vi "Modbus Message Loop.vi"(0 "Message Queues in":T2, 1 "PLC IP address":string="10.2.0.11", 3 "error in (no error)":errorcluster) -> (10 "error out":errorcluster)   [LabVIEW 2020, in "Modbus.lvlib"]
uses:
  Modbus.lvlib
  support/Message Queue/All Message Queues.ctl
  support/Message Queue/Message Cluster.ctl
  <vilib>/NI/Modbus Library/API/Master/Modbus Master.lvclass
  support/Message Queue/Enqueue Message (Single).vi
  <vilib>/NI/Modbus Library/API/Wrapper/Create TCP Master.vi
  support/Message Queue/Message Queue.lvlib
  <vilib>/NI/Modbus Library/API/Wrapper/API Main.lvlib
panel:
  in  "Loop Rate":u32=400
  out "size(s)":i32
  out "elements":T1[](array[typedef])
  out "Current State":string
  out "LDO Output Value":u32
  out "LDO Array 2":bool[](array[boolean])
  in  "Read States":bool
  out "States":string[](array[string])
  out "LDO Array 1":bool[](array[boolean])
  out "Loop Count":i32
  out "FV Output":bool[](array[boolean])
  out "Input Registers":u16[](array[numeric])
  # "Anybus: 192.168.0.50\nPLC: 192.168.0.20\n\nThis is available in the front HMI, e. IP and port. Useful for debugging and IP config change"
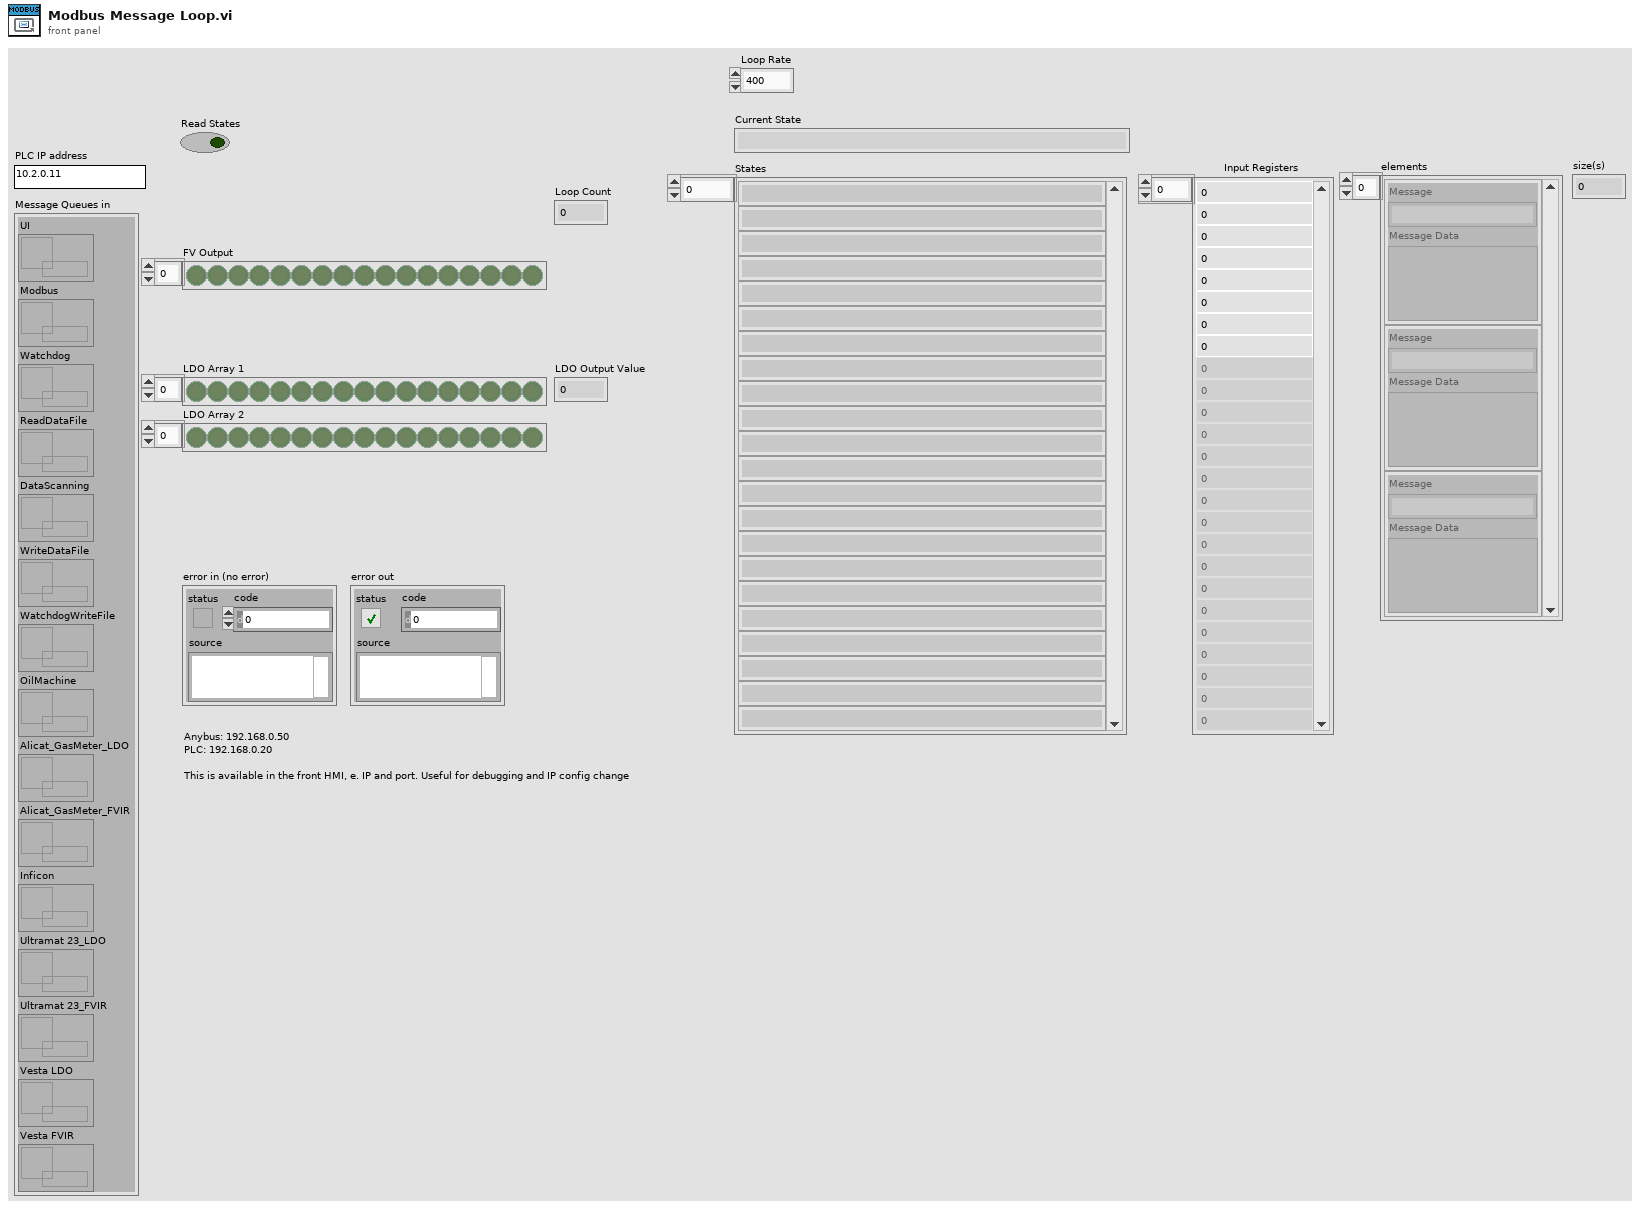
[diagram p1: front panel]
types:
  T1 = typedef "Message Queue.lvlib/Message Cluster.ctl" = cluster{"Message":string, "Message Data":variant}
  T2 = typedef "Message Queue.lvlib/All Message Queues.ctl" = cluster{"UI":refnum<queue>, "Modbus":refnum<queue>, "Watchdog":refnum<queue>, "ReadDataFile":refnum<queue>, "DataScanning":refnum<queue>, "WriteDataFile":refnum<queue>, "WatchdogWriteFile":refnum<queue>, "OilMachine":refnum<queue>, "Alicat_GasMeter_LDO":refnum<queue>, "Inficon":refnum<queue>, "Ultramat 23_LDO":refnum<queue>, "Alicat_GasMeter_FVIR":refnum<queue>, "Ultramat 23_FVIR":refnum<queue>, "Vesta LDO":refnum<queue>, "Vesta FVIR":refnum<queue>}
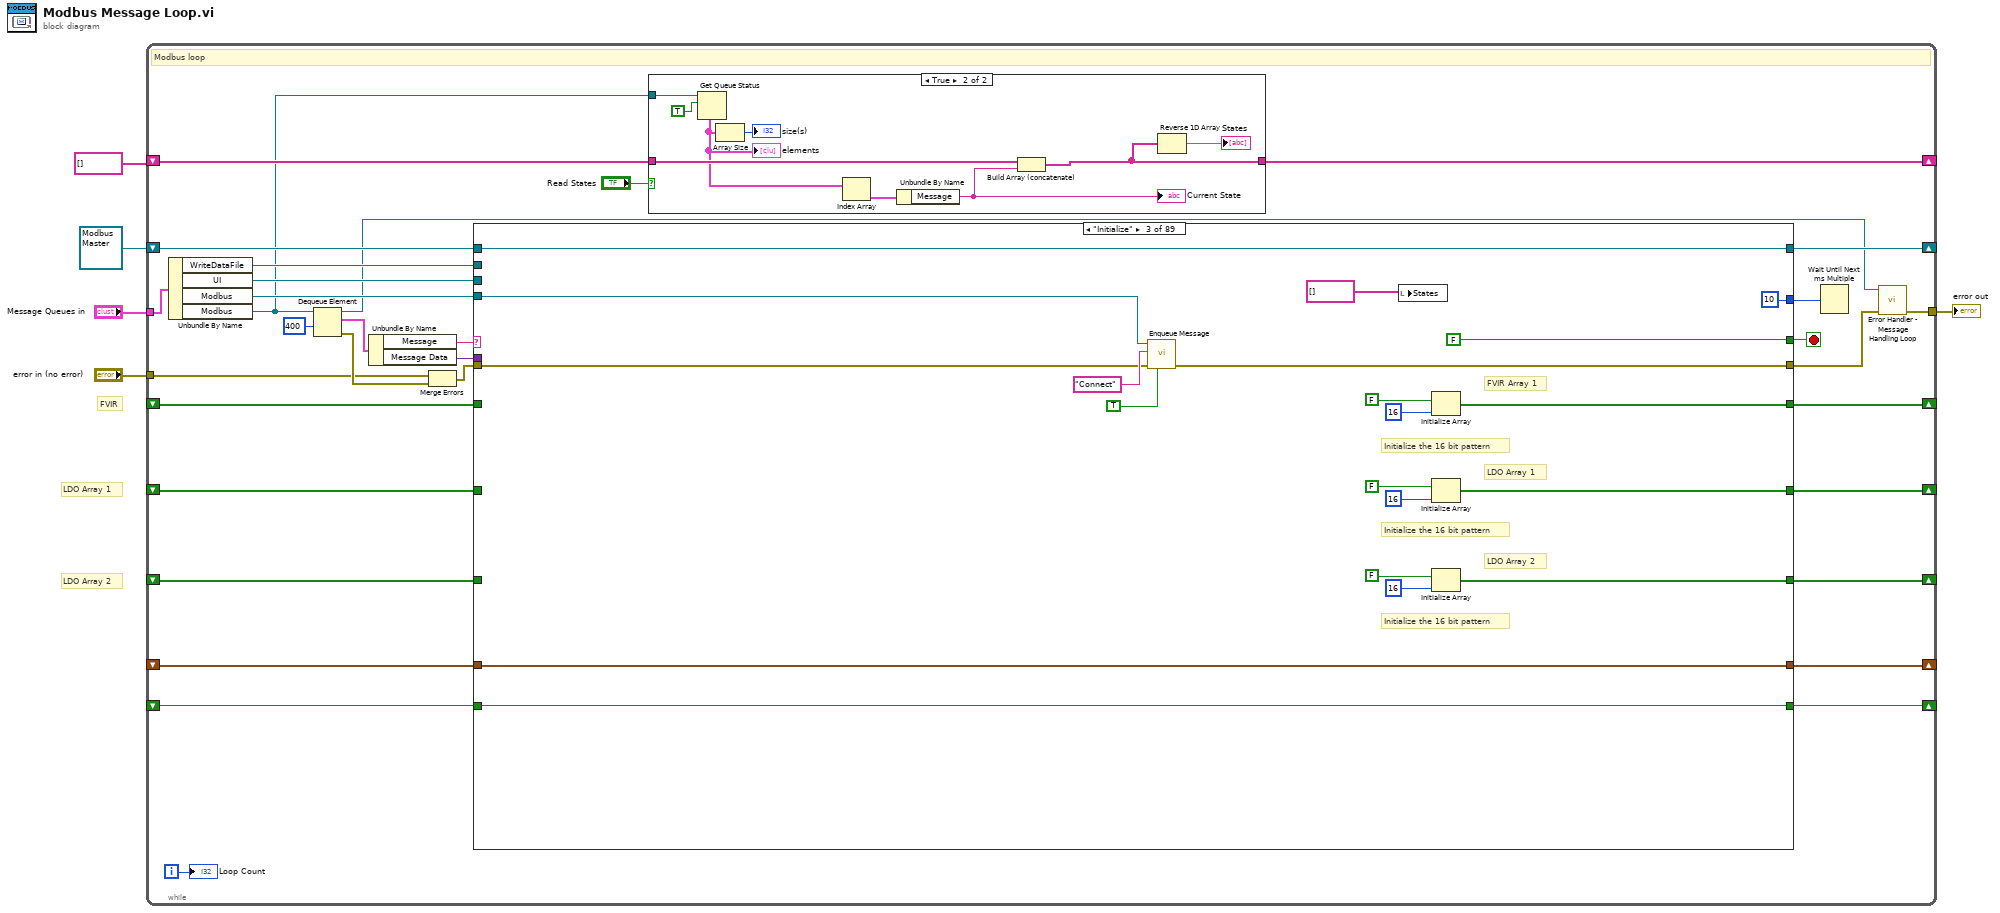
[diagram p0: block diagram]
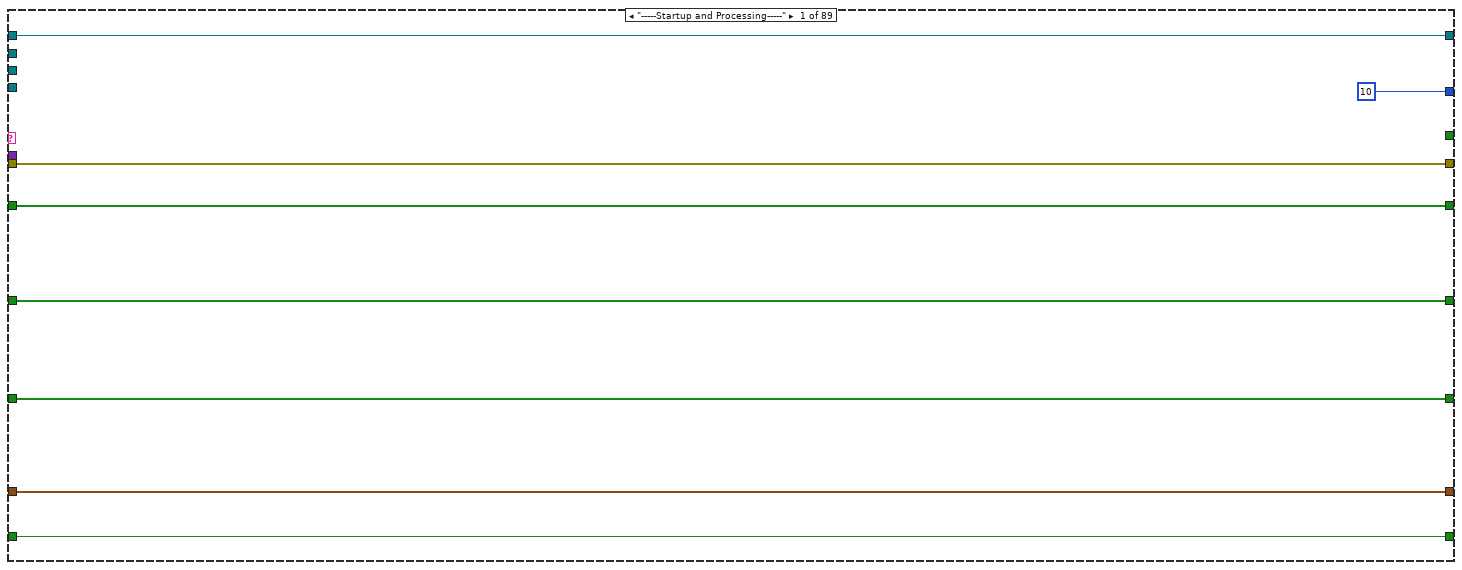
[diagram p3: hidden frame]
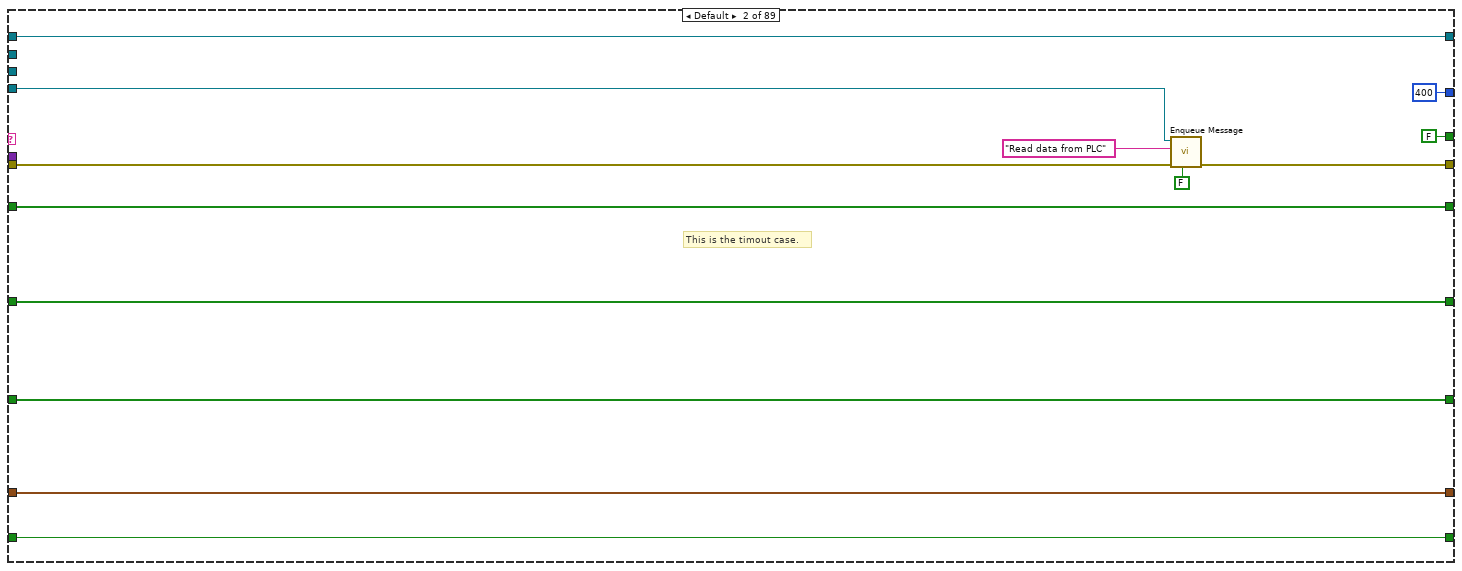
[diagram p4: hidden frame]
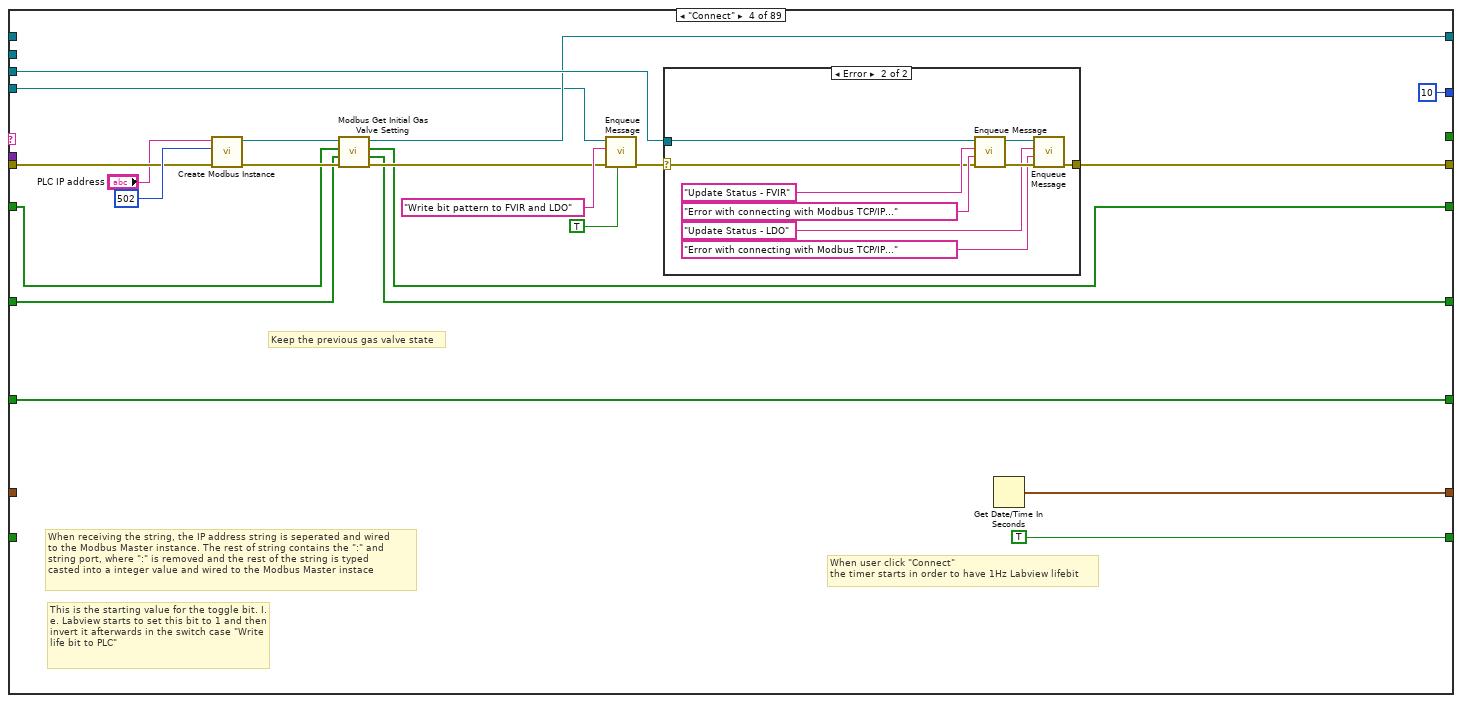
[diagram p5: hidden frame]
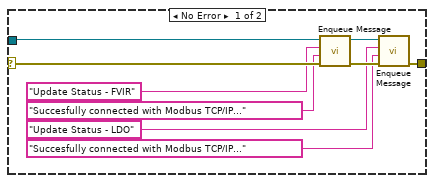
[diagram p6: hidden frame]
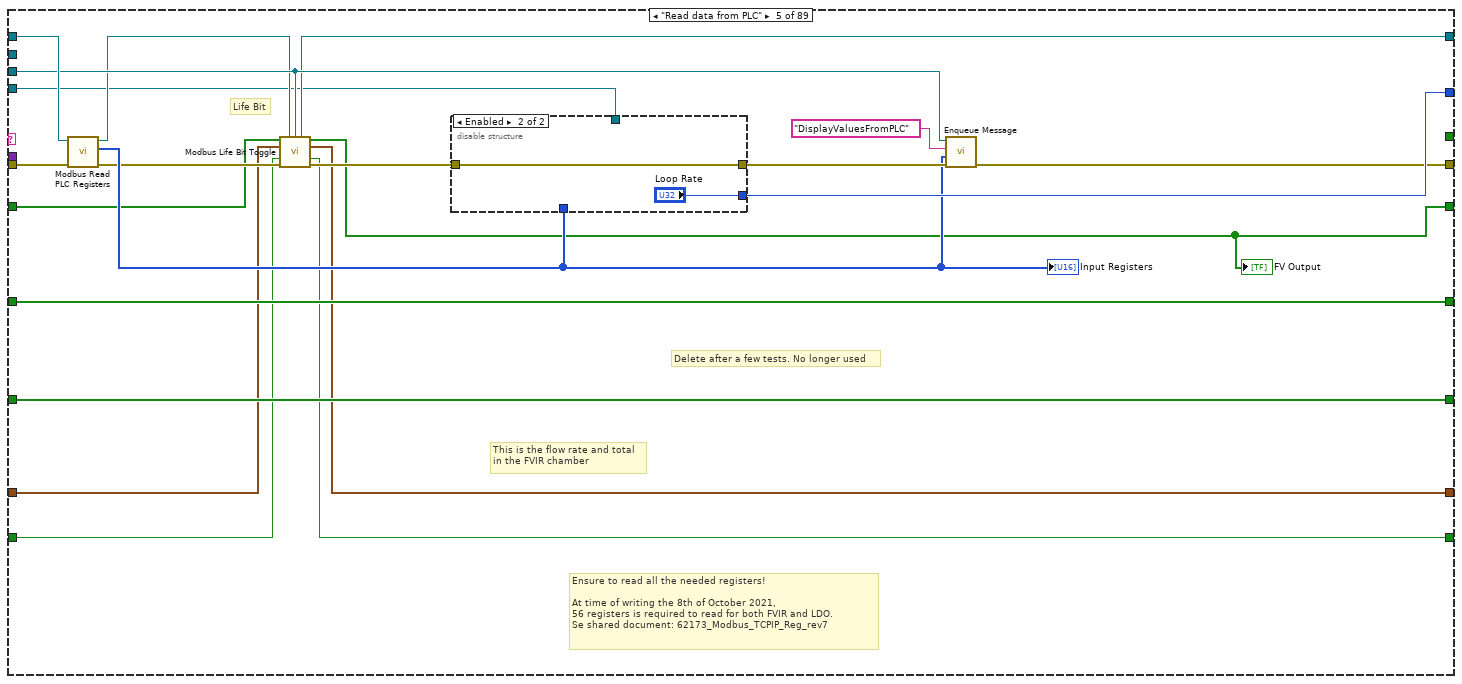
[diagram p7: hidden frame]
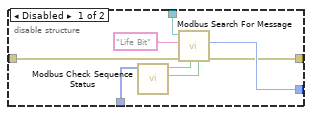
[diagram p8: hidden frame]
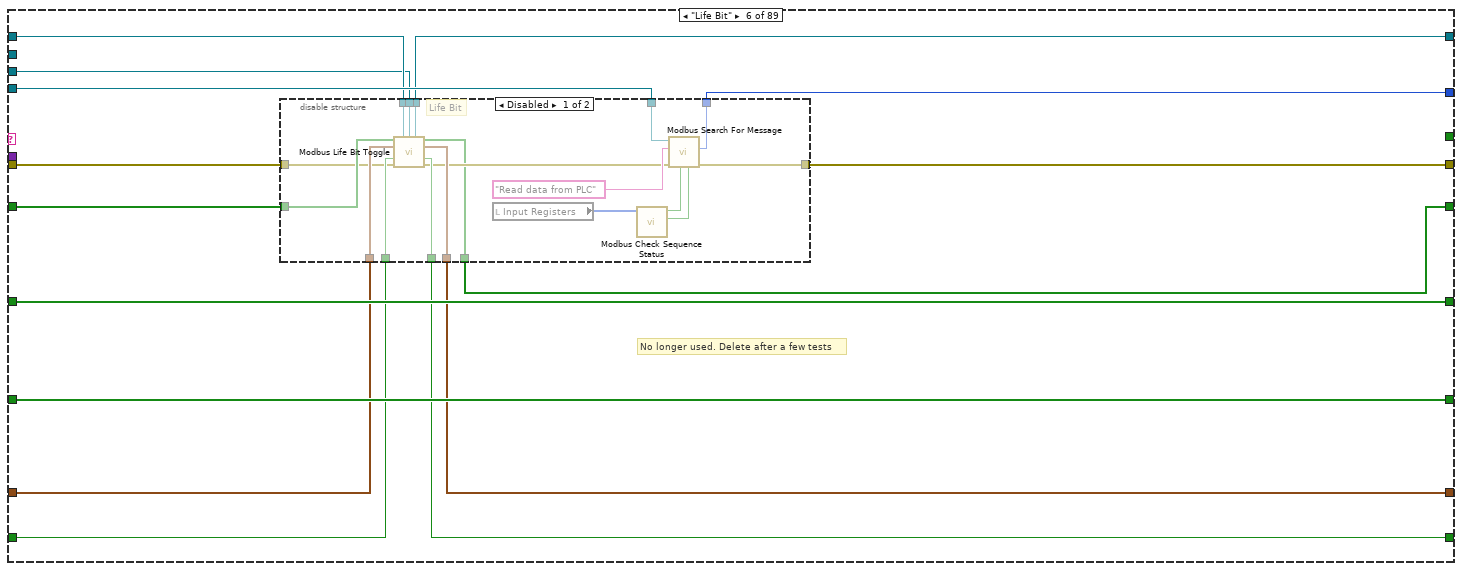
[diagram p9: hidden frame]
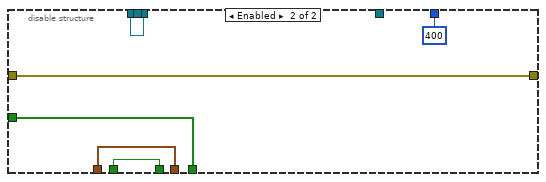
[diagram p10: hidden frame]
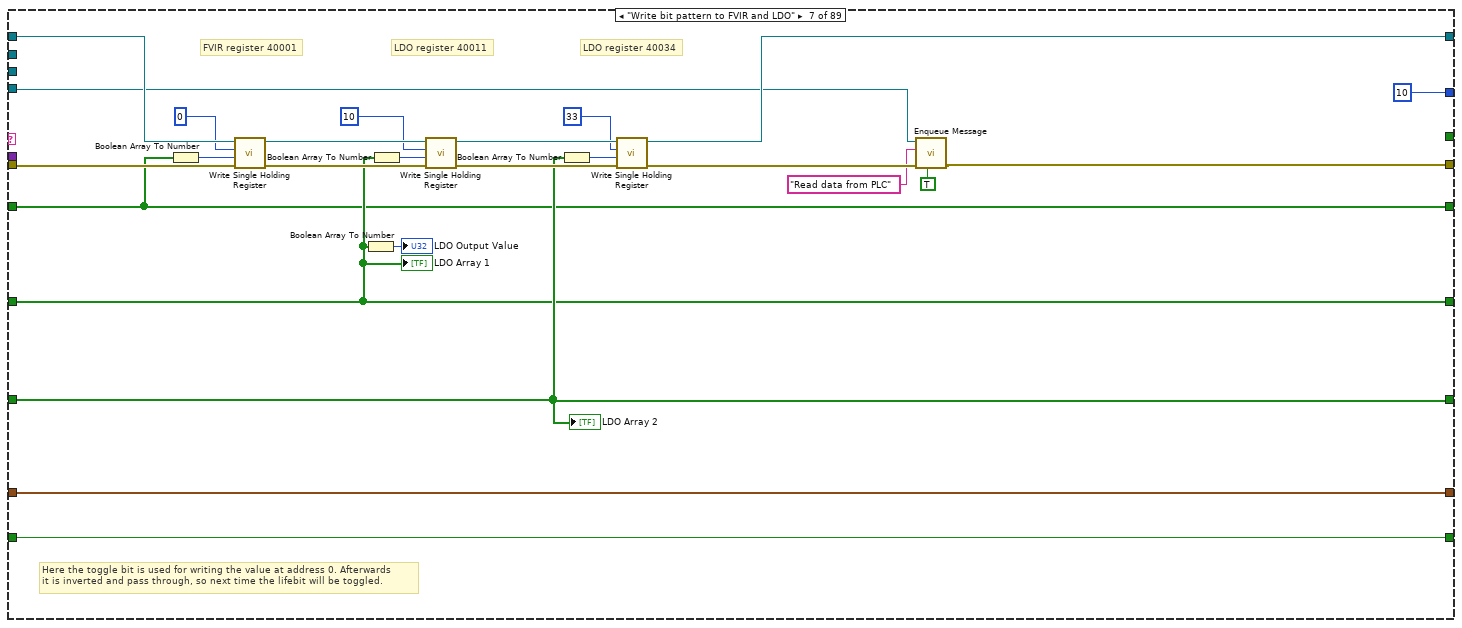
[diagram p11: hidden frame]
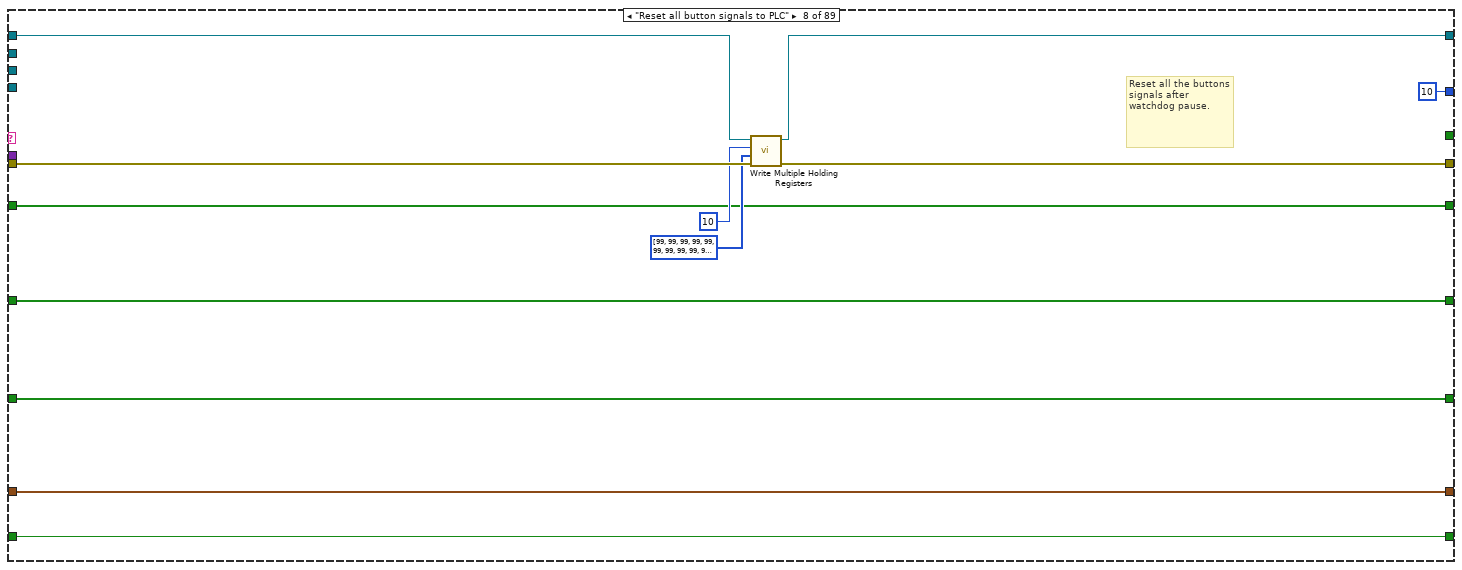
[diagram p12: hidden frame]
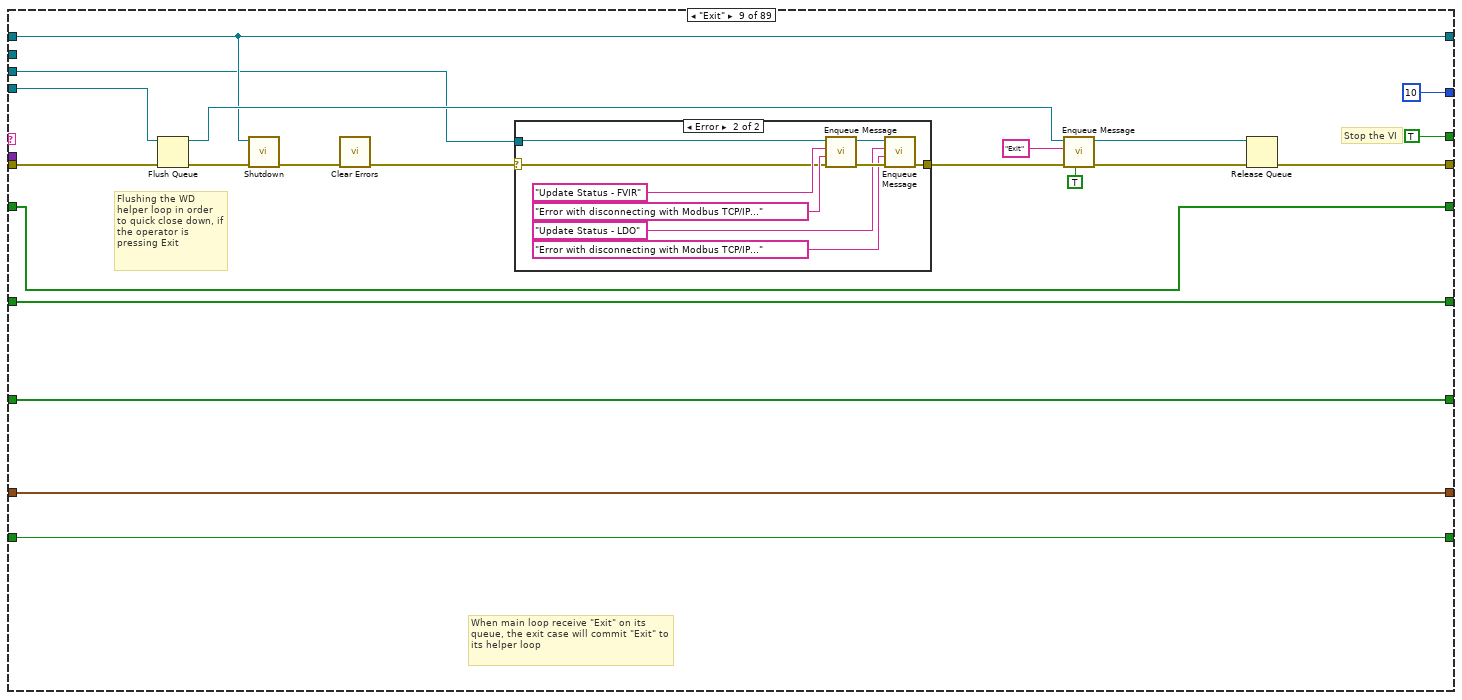
[diagram p13: hidden frame]
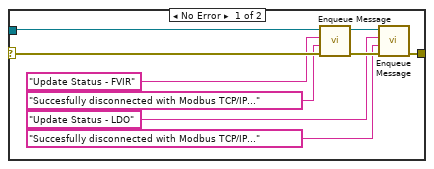
[diagram p14: hidden frame]
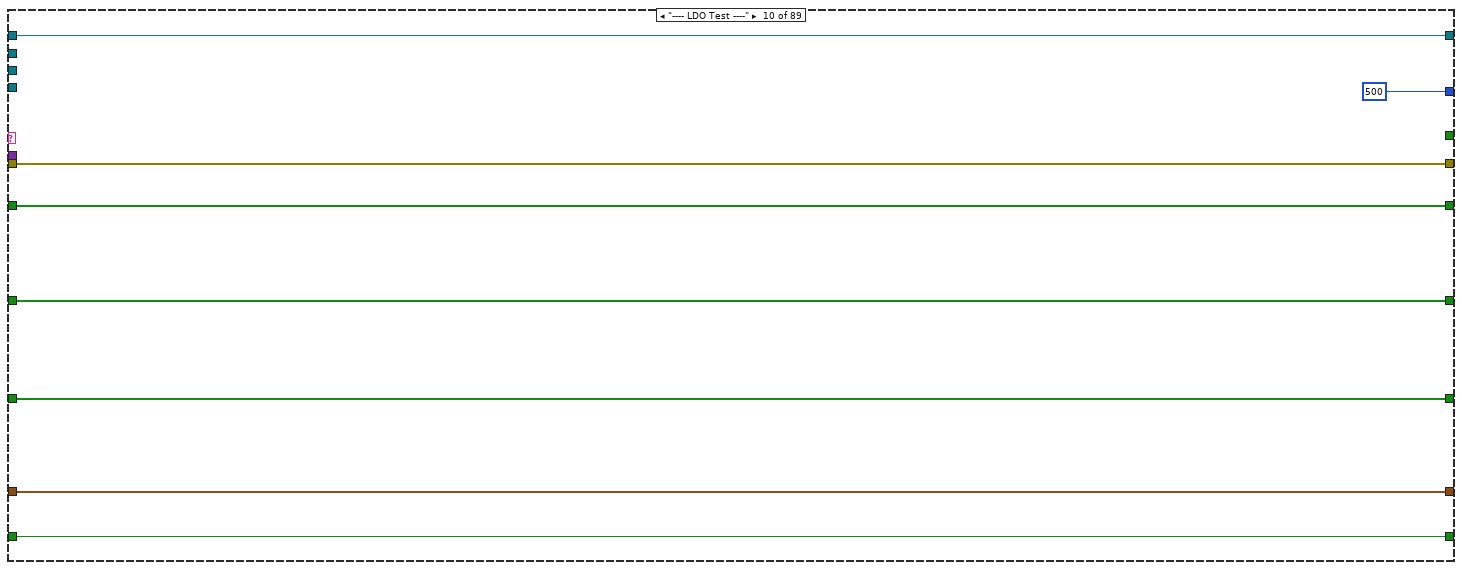
[diagram p15: hidden frame]
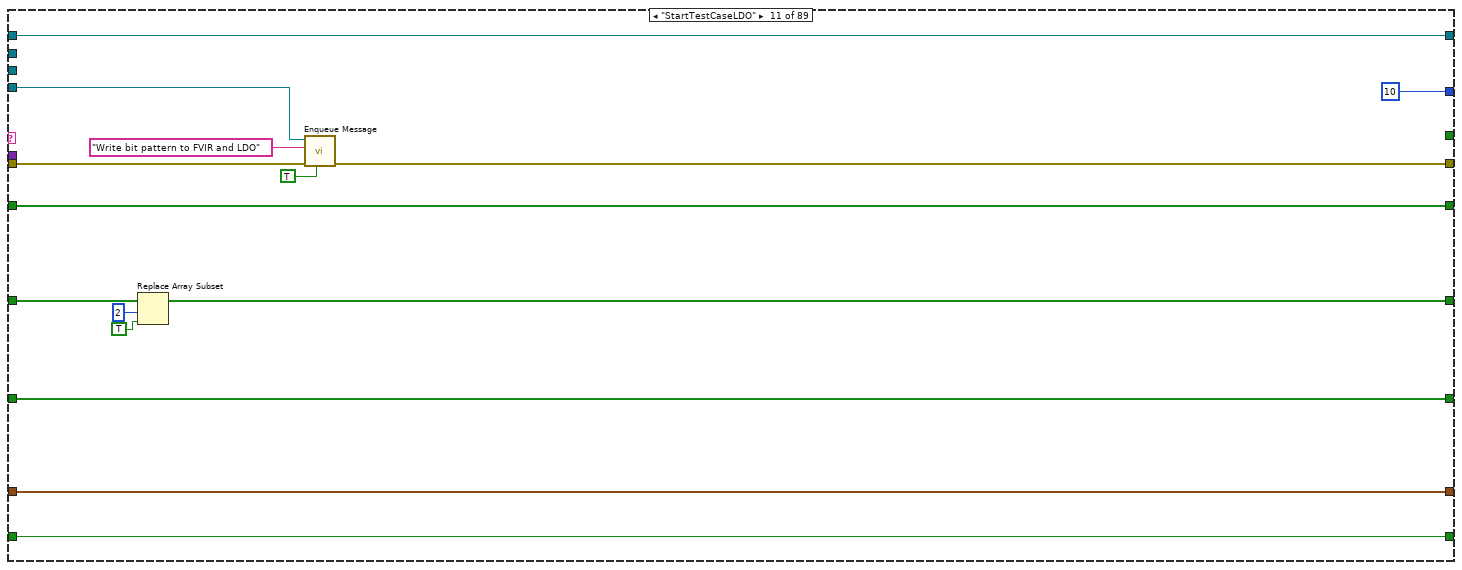
[diagram p16: hidden frame]
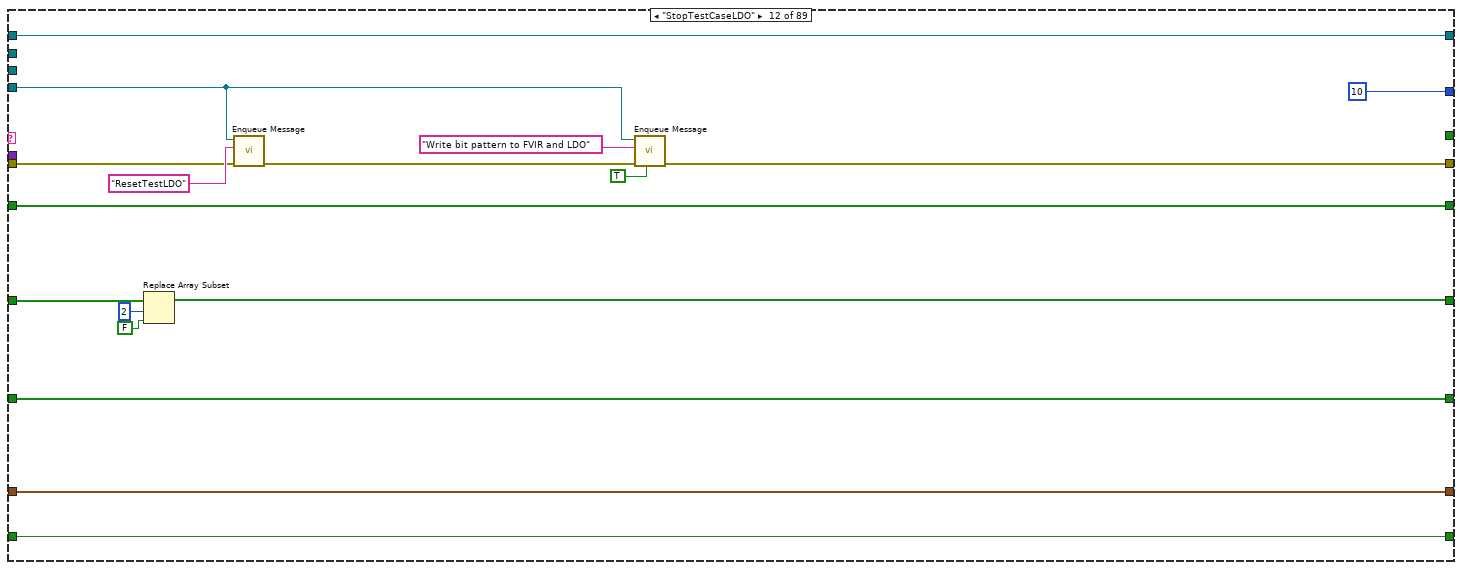
[diagram p17: hidden frame]
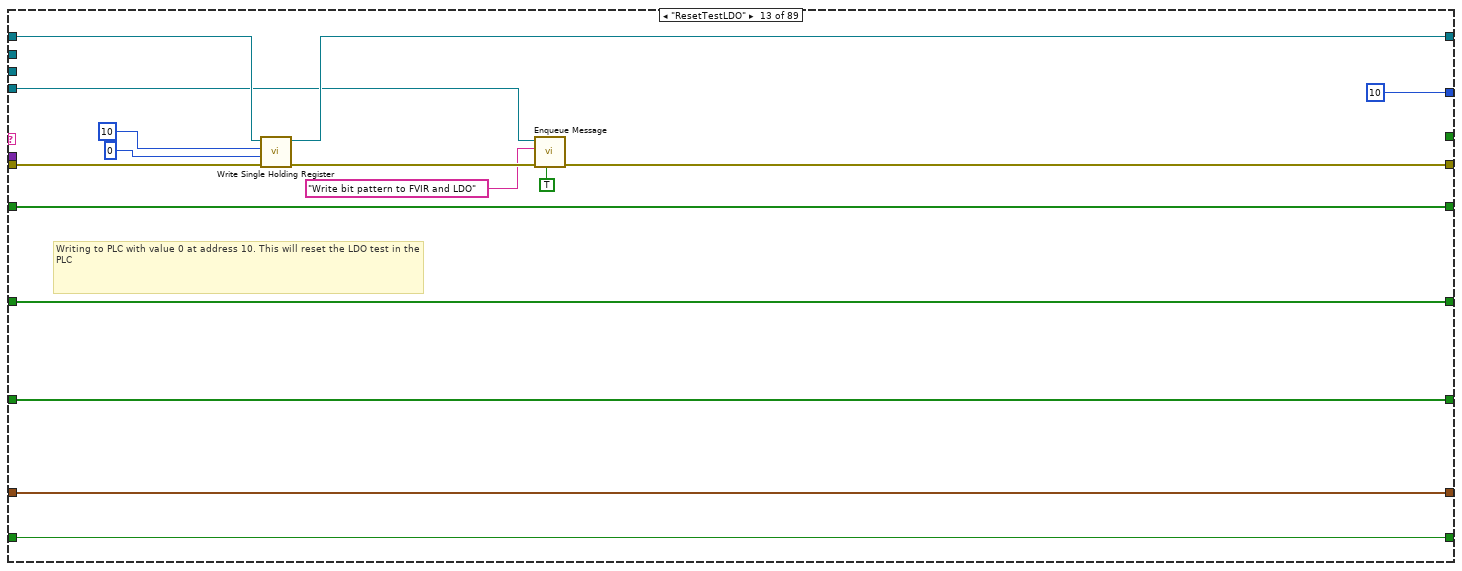
[diagram p18: hidden frame]
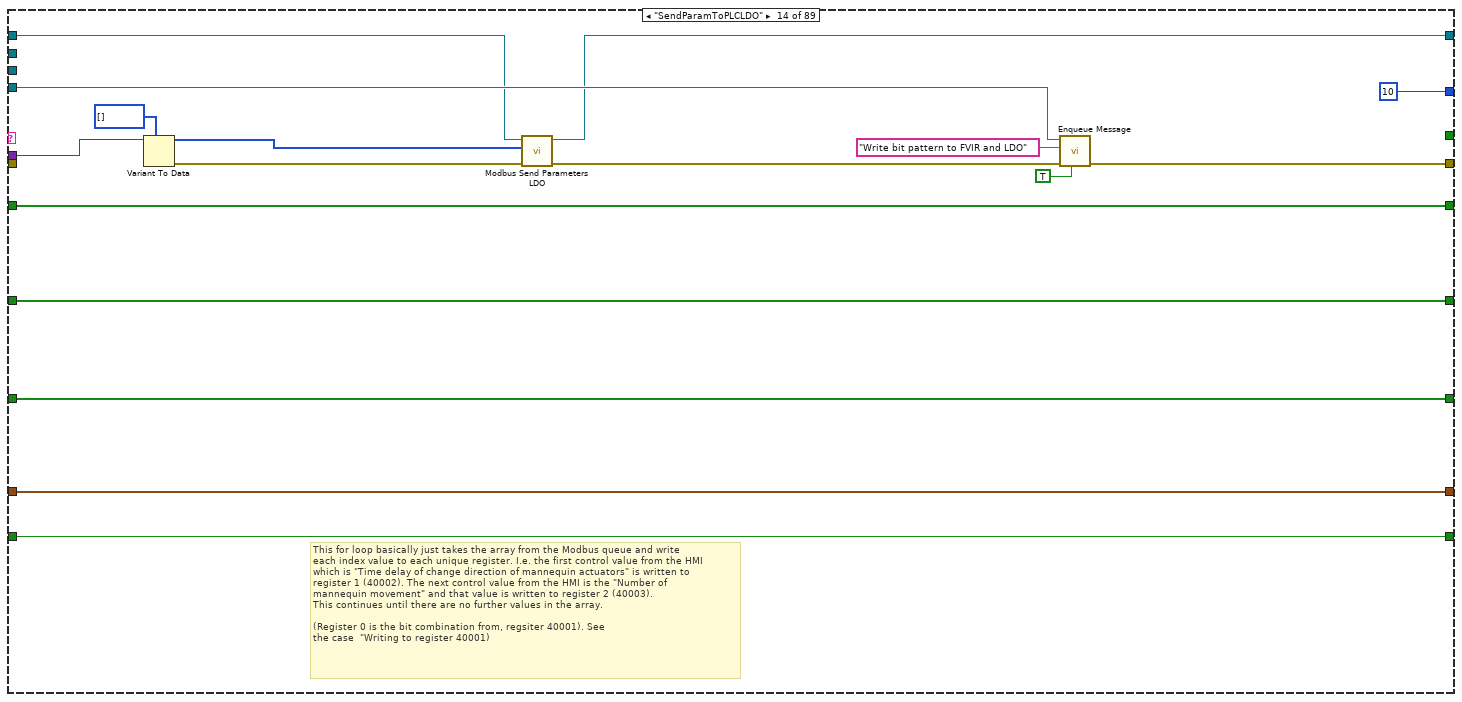
[diagram p19: hidden frame]
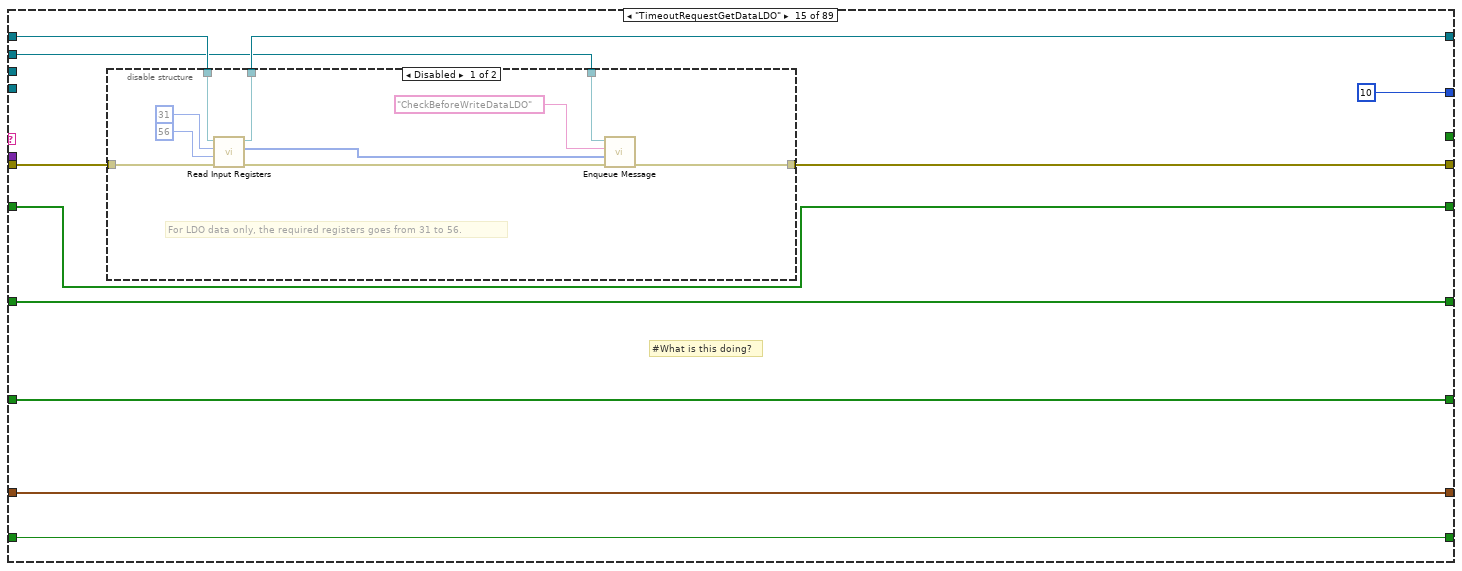
[diagram p20: hidden frame]
diagram:
  # "LDO Array 2"
  # "LDO Array 1"
  # "FVIR"
  n1 = while {
    tunnel: "Message Queues in" -> [w37]
    tunnel: [w36] -> w1
    tunnel: "error in (no error)" -> [w8]
    shift-right: [w34] -> _
    shift-left: refnum<class "Modbus Master.lvclass"> refnum ("Modbus Master") -> [w35]
    shift-right: [w32] -> _
    shift-left: _ -> [w31]
    shift-right: [w29] -> _
    shift-left: _ -> [w28]
    shift-right: [w26] -> _
    shift-left: _ -> [w25]
    shift-right: [w24] -> _
    shift-left: _ -> [w23]
    shift-right: [w20] -> _
    shift-left: string[] [] -> [w21]
    shift-right: [w18] -> _
    shift-left: _ -> [w17]
    i -> [w22]
    stop <- w38 stop-if-true
    # "Modbus loop"
    n2 = Unbundle By Name(w37) -> ("WriteDataFile"=w27:refnum<queue>, "UI"=w30:refnum<queue>, "Modbus"=w33:refnum<queue>, "Modbus"=w12:refnum<queue>)
    n3 = Dequeue Element(queue=w12, timeout in ms (-1)=400) -> (queue out=w11:refnum<queue>, element=w14:T1, error out=w13:errorcluster)  [unwired: 1 in, 1 out]
    n4 = Unbundle By Name(w14) -> ("Message"=w10:string, "Message Data"=w9:variant)
    n5 = Merge Errors(w8, w13) -> (w7:errorcluster)
    n6 = case shown="\"Initialize\"" w10 {
      tunnel: w7 -> [w51 w59 w78 w103 w145 w165 w216 w235 w247 w277 w293 w308 w330 _ w355 w381 w396 w411 w426 w441 w456 w471 w486 w497 w510 w536 w557 w578 w594 w615 w630 w645 w660 w675 w690 w705 w720 w733 w748 w760 w775 w790 w806 w820 w836 w851 w862 w879 w891 w913 _ w936 w970 w985 w1000 w1015 w1030 w1045 w1060 w1075 w1090 w1105 w1120 w1135 w1155 w1176 w1197 w1213 w1236 w1249 w1266 w1279 w1296 w1309 w1326 w1339 w1355 w1369 w1384 w1399 w1412 w1434 w1450 w1466 w1482 w1498 w1514 w1522 w1546]
      tunnel: [w51 w58 w77 w109 w129 w160 w202 w231 w240 w277 w296 w310 w322 w343 w353 w384 w399 w414 w429 w444 w459 w474 w489 w494 w509 w524 w549 w567 w588 w618 w633 w648 w663 w678 w693 w708 w723 w732 w747 w759 w774 w789 w807 w822 w837 w852 w862 w881 w886 w905 w926 w938 w973 w988 w1003 w1018 w1033 w1048 w1063 w1078 w1093 w1108 w1123 w1138 w1143 w1164 w1186 w1207 w1224 w1252 w1254 w1282 w1284 w1312 w1314 w1342 w1354 w1367 w1387 w1402 w1411 w1426 w1442 w1458 w1474 w1490 w1506 w1523 w1538] -> w15
      tunnel: [_ FALSE FALSE _ _ _ _ _ TRUE _ _ _ _ _ _ _ _ _ _ _ _ _ _ _ _ _ _ _ _ _ _ _ _ _ _ _ _ _ _ _ _ _ _ _ _ _ _ _ _ _ _ _ _ _ _ _ _ _ _ _ _ _ _ _ _ _ _ _ _ _ _ _ _ _ _ _ _ _ _ _ _ _ _ _ _ _ _ _ _] -> w38
      tunnel: w35 -> [w52 w65 w89 _ w144 w164 w223 w233 w243 w276 w294 w313 w328 w341 w358 w382 w397 w412 w427 w442 w457 w472 w487 w502 w517 w529 w553 w571 w592 w616 w631 w646 w661 w676 w691 w706 w721 w731 w746 w758 w773 w788 w802 w817 w832 w847 w863 w880 w897 w911 w924 w942 w971 w986 w1001 w1016 w1031 w1046 w1061 w1076 w1091 w1106 w1121 w1136 w1148 w1169 w1190 w1211 w1237 w1250 w1267 w1280 w1297 w1310 w1327 w1340 w1353 w1366 w1385 w1400 w1410 w1432 w1448 w1464 w1480 w1496 w1512 w1529 w1544]
      tunnel: [w52 w65 w89 w98 w137 w163 w212 w234 w243 w276 w294 w313 w329 w340 w357 w382 w397 w412 w427 w442 w457 w472 w487 w502 w517 w528 w552 w570 w591 w616 w631 w646 w661 w676 w691 w706 w721 w731 w746 w758 w773 w788 w802 w817 w832 w847 w863 w880 w897 w912 w923 w941 w971 w986 w1001 w1016 w1031 w1046 w1061 w1076 w1091 w1106 w1121 w1136 w1147 w1168 w1189 w1210 w1237 w1250 w1267 w1280 w1297 w1310 w1327 w1340 w1353 w1366 w1385 w1400 w1410 w1433 w1449 w1465 w1481 w1497 w1513 w1530 w1545] -> w34
      tunnel: w33 -> [_ w57 w70 w90 w132 w172 w201 _ w246 _ w297 w298 w325 w347 _ w385 w400 w415 w430 w445 w460 w475 w490 w498 w511 w526 w550 w566 w587 w619 w634 w649 w664 w679 w694 w709 w724 w734 w749 w761 w776 w791 w805 w821 w835 w850 _ w882 w883 w908 w930 _ w974 w989 w1004 w1019 w1034 w1049 w1064 w1079 w1094 w1109 w1124 w1139 w1145 w1166 w1185 w1206 w1231 w1253 w1261 w1283 w1291 w1313 w1321 w1343 w1356 w1368 w1388 w1403 w1413 w1429 w1445 w1461 w1477 w1493 w1509 w1526 w1541]
      tunnel: w9 -> [_ _ _ _ _ _ _ _ _ _ _ _ _ w345 _ _ _ _ _ _ _ _ _ _ _ w535 w556 w577 w593 _ _ _ _ _ _ _ _ _ _ _ _ _ _ _ _ _ _ _ _ _ w928 w935 _ _ _ _ _ _ _ _ _ _ _ _ w1154 w1175 w1196 w1212 _ _ _ _ _ _ _ _ _ _ _ _ _ _ _ _ _ _ _ _ _]
      tunnel: [w56 w69 w85 w96 w131 w162 w205 w229 w252 w282 w288 w306 w321 w337 w356 w376 w391 w406 w421 w436 w451 w466 w481 w505 w520 w541 w562 w583 w604 w610 w625 w640 w655 w670 w685 w700 w715 w739 w754 w769 w784 w799 w814 w829 w844 w859 w867 w876 w894 w904 w920 w940 w967 w982 w997 w1012 w1027 w1042 w1057 w1072 w1087 w1102 w1117 w1132 w1160 w1181 w1202 w1223 w1233 w1246 w1263 w1276 w1293 w1306 w1323 w1336 w1346 w1361 w1381 w1396 w1407 w1425 w1441 w1457 w1473 w1489 w1505 w1521 w1537] -> w32
      tunnel: w31 -> [w56 w69 _ w97 w136 w166 w205 w229 w252 w282 w288 w306 w321 w337 w356 w376 w391 w406 w421 w436 w451 w466 w481 w505 w520 w541 w562 w583 w604 w610 w625 w640 w655 w670 w685 w700 w715 w739 w754 w769 w784 w799 w814 w829 w844 w859 w867 w877 w895 w904 w920 w940 w968 w983 w998 w1013 w1028 w1043 w1058 w1073 w1088 w1103 w1118 w1133 w1160 w1181 w1202 w1223 w1234 w1247 w1264 w1277 w1294 w1307 w1324 w1337 w1347 w1362 w1382 w1397 w1408 w1425 w1441 w1457 w1473 w1489 w1505 w1521 w1537]
      tunnel: w30 -> [_ _ _ w110 w139 w161 _ _ w237 _ _ _ _ _ _ _ _ _ _ _ _ _ _ _ _ _ _ _ _ _ _ _ _ _ _ _ _ _ _ _ _ _ _ _ _ _ _ _ _ _ _ _ _ _ _ _ _ _ _ _ _ _ _ _ _ _ _ _ _ _ _ _ _ _ _ _ _ _ _ _ _ _ _ _ _ _ _ _ _]
      tunnel: [w55 w68 w82 w94 w149 w173 w207 w228 w251 w281 w289 w304 w320 w336 w354 w377 w392 w407 w422 w437 w452 w467 w482 w495 w512 w540 w561 w582 w603 w611 w626 w641 w656 w671 w686 w701 w716 w735 w750 w763 w778 w793 w813 w828 w843 w858 w866 w874 w890 w903 w919 w939 w965 w980 w995 w1010 w1025 w1040 w1055 w1070 w1085 w1100 w1115 w1130 w1159 w1180 w1201 w1222 w1230 w1244 w1260 w1274 w1290 w1304 w1320 w1334 w1350 w1373 w1379 w1394 w1406 w1424 w1440 w1456 w1472 w1488 w1504 w1520 w1536] -> w29
      tunnel: w28 -> [w55 w68 _ w95 w149 w173 w207 w228 w251 w281 w290 w305 w320 w336 w354 w378 w393 w408 w423 w438 w453 w468 w483 w496 w513 w540 w561 w582 w603 w612 w627 w642 w657 w672 w687 w702 w717 w736 w751 w764 w779 w794 w813 w828 w843 w858 w866 w874 w890 w903 w919 w939 w965 w980 w995 w1010 w1025 w1040 w1055 w1070 w1085 w1100 w1115 w1130 w1159 w1180 w1201 w1222 w1230 w1244 w1260 w1274 w1290 w1304 w1320 w1334 w1350 w1373 w1379 w1394 w1406 w1424 w1440 w1456 w1472 w1488 w1504 w1520 w1536]
      tunnel: w27 -> [_ _ _ _ _ _ _ _ _ _ _ _ _ _ w352 _ _ _ _ _ _ _ _ _ _ _ _ _ _ _ _ _ _ _ _ _ _ _ _ _ _ _ _ _ _ _ _ _ _ _ _ w937 _ _ _ _ _ _ _ _ _ _ _ _ _ _ _ _ _ _ _ _ _ _ _ _ _ _ _ _ _ _ _ _ _ _ _ _ _]
      tunnel: [w54 w67 w81 w106 w134 w167 w204 w227 w250 w280 w287 w303 w319 w335 w351 w375 w390 w405 w420 w435 w450 w465 w480 w504 w519 w539 w560 w581 w602 w609 w624 w639 w654 w669 w684 w699 w714 w738 w753 w768 w783 w798 w812 w827 w842 w857 w865 w872 w889 w902 w918 w934 w964 w979 w994 w1009 w1024 w1039 w1054 w1069 w1084 w1099 w1114 w1129 w1158 w1179 w1200 w1221 w1229 w1243 w1259 w1273 w1289 w1303 w1319 w1333 w1358 w1372 w1378 w1393 w1418 w1423 w1439 w1455 w1471 w1487 w1503 w1519 w1535] -> w26
      tunnel: w25 -> [w54 w67 w81 _ w135 w169 w204 w227 w250 w280 w287 w303 w319 w335 w351 w375 w390 w405 w420 w435 w450 w465 w480 w504 w519 w539 w560 w581 w602 w609 w624 w639 w654 w669 w684 w699 w714 w738 w753 w768 w783 w798 w812 w827 w842 w857 w865 w872 w889 w902 w918 w934 w964 w979 w994 w1009 w1024 w1039 w1054 w1069 w1084 w1099 w1114 w1129 w1158 w1179 w1200 w1221 w1229 w1243 w1259 w1273 w1289 w1303 w1319 w1333 w1358 w1372 w1378 w1393 w1418 w1423 w1439 w1455 w1471 w1487 w1503 w1519 w1535]
      tunnel: [w53 w66 w80 TRUE w130 w168 w203 w226 w249 w279 w286 w302 w318 w334 w350 w374 w389 w404 w419 w434 w449 w464 w479 w503 w518 w538 w559 w580 w601 w608 w623 w638 w653 w668 w683 w698 w713 w737 w752 w767 w782 w797 w811 w826 w841 w856 w864 w871 w888 w901 w917 w933 w963 w978 w993 w1008 w1023 w1038 w1053 w1068 w1083 w1098 w1113 w1128 w1157 w1178 w1199 w1220 w1228 w1242 w1258 w1272 w1288 w1302 w1318 w1332 w1357 w1371 w1377 w1392 w1417 w1422 w1438 w1454 w1470 w1486 w1502 w1518 w1534] -> w24
      tunnel: w23 -> [w53 w66 w80 _ w133 w170 w203 w226 w249 w279 w286 w302 w318 w334 w350 w374 w389 w404 w419 w434 w449 w464 w479 w503 w518 w538 w559 w580 w601 w608 w623 w638 w653 w668 w683 w698 w713 w737 w752 w767 w782 w797 w811 w826 w841 w856 w864 w871 w888 w901 w917 w933 w963 w978 w993 w1008 w1023 w1038 w1053 w1068 w1083 w1098 w1113 w1128 w1157 w1178 w1199 w1220 w1228 w1242 w1258 w1272 w1288 w1302 w1318 w1332 w1357 w1371 w1377 w1392 w1417 w1422 w1438 w1454 w1470 w1486 w1502 w1518 w1534]
      tunnel: [w50 w62 w74 w93 w148 w174 w209 w225 w239 w278 w285 w301 w317 w333 w349 w373 w388 w403 w418 w433 w448 w463 w478 w493 w508 w523 w548 w565 w586 w607 w622 w637 w652 w667 w682 w697 w712 w730 w745 w757 w772 w787 w803 w819 w833 w848 w861 w870 w887 w900 w916 w932 w962 w977 w992 w1007 w1022 w1037 w1052 w1067 w1082 w1097 w1112 w1127 w1142 w1163 w1184 w1205 w1227 w1241 w1257 w1271 w1287 w1301 w1317 w1331 w1352 w1365 w1376 w1391 w1409 w1421 w1437 w1453 w1469 w1485 w1501 w1517 w1533] -> w18
      tunnel: w17 -> [w50 w62 _ w93 w148 w174 w209 w225 w239 w278 w285 w301 w317 w333 w349 w373 w388 w403 w418 w433 w448 w463 w478 w493 w508 w523 w548 w565 w586 w607 w622 w637 w652 w667 w682 w697 w712 w730 w745 w757 w772 w787 w804 w818 w834 w849 w861 w870 w887 w900 w916 w932 w962 w977 w992 w1007 w1022 w1037 w1052 w1067 w1082 w1097 w1112 w1127 w1142 w1163 w1184 w1205 w1227 w1241 w1257 w1271 w1287 w1301 w1317 w1331 w1352 w1365 w1376 w1391 w1409 w1421 w1437 w1453 w1469 w1485 w1501 w1517 w1533]
      tunnel: [u32 10 ("millisecond multiple") u32 400 ("millisecond multiple") u32 10 ("millisecond multiple") u32 10 ("millisecond multiple") w146 w171 u32 10 ("millisecond multiple") u32 10 ("millisecond multiple") u32 10 ("millisecond multiple") u32 500 ("millisecond multiple") u32 10 ("millisecond multiple") u32 10 ("millisecond multiple") u32 10 ("millisecond multiple") u32 10 ("millisecond multiple") u32 10 ("millisecond multiple") u32 10 ("millisecond multiple") u32 10 ("millisecond multiple") u32 10 ("millisecond multiple") u32 10 ("millisecond multiple") u32 10 ("millisecond multiple") u32 10 ("millisecond multiple") u32 10 ("millisecond multiple") u32 10 ("millisecond multiple") u32 10 ("millisecond multiple") u32 10 ("millisecond multiple") u32 10 ("millisecond multiple") u32 10 ("millisecond multiple") u32 10 ("millisecond multiple") u32 10 ("millisecond multiple") u32 10 ("millisecond multiple") u32 10 ("millisecond multiple") u32 10 ("millisecond multiple") u32 10 ("millisecond multiple") u32 10 ("millisecond multiple") u32 10 ("millisecond multiple") u32 10 ("millisecond multiple") u32 10 ("millisecond multiple") u32 10 ("millisecond multiple") u32 10 ("millisecond multiple") u32 10 ("millisecond multiple") u32 10 ("millisecond multiple") u32 10 ("millisecond multiple") u32 10 ("millisecond multiple") u32 10 ("millisecond multiple") u32 10 ("millisecond multiple") u32 10 ("millisecond multiple") u32 10 ("millisecond multiple") u32 10 ("millisecond multiple") u32 10 ("millisecond multiple") u32 10 ("millisecond multiple") u32 10 ("millisecond multiple") u32 10 ("millisecond multiple") u32 10 ("millisecond multiple") u32 10 ("millisecond multiple") u32 10 ("millisecond multiple") u32 10 ("millisecond multiple") u32 10 ("millisecond multiple") u32 10 ("millisecond multiple") u32 10 ("millisecond multiple") u32 10 ("millisecond multiple") u32 10 ("millisecond multiple") u32 10 ("millisecond multiple") u32 10 ("millisecond multiple") u32 10 ("millisecond multiple") u32 10 ("millisecond multiple") u32 10 ("millisecond multiple") u32 10 ("millisecond multiple") u32 10 ("millisecond multiple") u32 10 ("millisecond multiple") u32 10 ("millisecond multiple") u32 10 ("millisecond multiple") u32 10 ("millisecond multiple") u32 10 ("millisecond multiple") u32 10 ("millisecond multiple") u32 10 ("millisecond multiple") u32 10 ("millisecond multiple") u32 10 ("millisecond multiple") u32 10 ("millisecond multiple") u32 10 ("millisecond multiple") u32 10 ("millisecond multiple") u32 10 ("millisecond multiple") u32 10 ("millisecond multiple") u32 10 ("millisecond multiple") u32 10 ("millisecond multiple") u32 10 ("millisecond multiple") u32 10 ("millisecond multiple") u32 10 ("millisecond multiple") u32 10 ("millisecond multiple") u32 10 ("millisecond multiple")] -> w16
      frame "-----Startup and Processing-----" {
      }
      frame Default {
        # "This is the timout case."
        n7 = call-poly "Enqueue Message.vi"("Priority Message? (F)"=FALSE, "error in (no error)"=w59, "Message"="Read data from PLC", "Message Queue"=w57) -> ("error out"=w58:errorcluster)  [unwired: 6 in, 1 out]
      }
      frame "Initialize" {
        # "LDO Array 2"
        # "Initialize the 16 bit pattern"
        # "LDO Array 1"
        # "FVIR Array 1"
        # "Initialize the 16 bit pattern"
        # "Initialize the 16 bit pattern"
        n8 = call-poly "Enqueue Message.vi"("Priority Message? (F)"=TRUE, "error in (no error)"=w78, "Message"="Connect", "Message Queue"=w70) -> ("error out"=w77:errorcluster)  [unwired: 6 in, 1 out]
        n9 = local write "States"(string[] []) -> ()
        n10 = Initialize Array(FALSE, 16 ("dimension size")) -> (w85:bool[])
        n11 = Initialize Array(FALSE, 16 ("dimension size")) -> (w82:bool[])
        n12 = Initialize Array(FALSE, 16 ("dimension size")) -> (w74:bool[])
      }
      frame "Connect" {
        # "Keep the previous gas valve state"
        # "When user click \"Connect\"\nthe timer starts in order to have 1Hz Labview lifebit"
        # "When receiving the string, the IP address string is seperated and wired\nto the Modbus Master instance. The rest of string contains the \":\" and\nstring port, where \":\" is removed and the rest of the string is typed \ncasted into a integer value and wired to the Modbus Master instace"
        # "This is the starting value for the toggle bit. I.e. Labview starts to set this bit to 1 and then invert it afterwards in the switch case \"Write life bit to PLC\""
        n13 = call-poly <vilib>:"Create Modbus Instance.vi"("error in"=w103, "port (502)"=u16 502 ("Port"), "address"="PLC IP address") -> ("error out"=w101:errorcluster, "TCP master instance"=w99:refnum<class "Modbus Master.lvclass">)  [unwired: 7 in]
        n14 = call "Modbus Get Initial Gas Valve Setting.vi"("error in (no error)"=w101, "LDO Input"=w95, "FVIR Input"=w97, "Modbus Master in"=w99) -> ("error out"=w100:errorcluster, "LDO Output"=w94:bool[], "FVIR Output"=w96:bool[], "Modbus Master out"=w98:refnum<class "Modbus Master.lvclass">)  [unwired: 4 in]
        n15 = call-poly "Enqueue Message.vi"("Priority Message? (F)"=TRUE, "error in (no error)"=w100, "Message"="Write bit pattern to FVIR and LDO", "Message Queue"=w90) -> ("error out"=w107:errorcluster)  [unwired: 6 in, 1 out]
        n16 = case shown="Error" w107 {
          selector: w107 -> [w119 w122]
          tunnel: w110 -> [w111 w120]
          tunnel: [w117 w121] -> w109
          frame No Error {
            n17 = call-poly "Enqueue Message.vi"("error in (no error)"=w119, "Message Data"="Succesfully connected with Modbus TCP/IP..." ("Acquiring and Logging..."), "Message"="Update Status - FVIR", "Message Queue"=w111) -> ("error out"=w118:errorcluster, "dup Message Queue"=w116:refnum<queue>)  [unwired: 6 in]
            n18 = call-poly "Enqueue Message.vi"("error in (no error)"=w118, "Message Data"="Succesfully connected with Modbus TCP/IP..." ("Acquiring and Logging..."), "Message"="Update Status - LDO", "Message Queue"=w116) -> ("error out"=w117:errorcluster)  [unwired: 6 in, 1 out]
          }
          frame Error {
            n19 = call-poly "Enqueue Message.vi"("error in (no error)"=w122, "Message Data"="Error with connecting with Modbus TCP/IP..." ("Acquiring and Logging..."), "Message"="Update Status - FVIR", "Message Queue"=w120) -> ("error out"=w128:errorcluster, "dup Message Queue"=w127:refnum<queue>)  [unwired: 6 in]
            n20 = call-poly "Enqueue Message.vi"("error in (no error)"=w128, "Message Data"="Error with connecting with Modbus TCP/IP..." ("Acquiring and Logging..."), "Message"="Update Status - LDO", "Message Queue"=w127) -> ("error out"=w121:errorcluster)  [unwired: 6 in, 1 out]
          }
        }
        n21 = Get Date/Time In Seconds() -> (seconds since 1Jan1904=w106:timestamp)
      }
      frame "Read data from PLC" {
        # "Delete after a few tests. No longer used"
        # "Life Bit"
        # "This is the flow rate and total\nin the FVIR chamber"
        # "Ensure to read all the needed registers! \n\nAt time of writing the 8th of October 2021, \n56 registers is required to read for both FVIR and LDO. \nSe shared document: 62173_Modbus_TCPIP_Reg_rev7"
        n22 = call "Modbus Read PLC Registers.vi"("error in (no error)"=w145, "Modbus Master in"=w144) -> ("error out"=w141:errorcluster, "Input Registers"=w142:u16[], "Modbus Master out"=w138:refnum<class "Modbus Master.lvclass">)  [unwired: 7 in]
        "Input Registers" <- w142
        n23 = call "Modbus Life Bit Toggle.vi"("FVIR Boolean Array Input"=w136, "Modbus master in"=w138, "UI"=w139, "seconds since 1Jan1904 in"=w135, "Toggle Input"=w133, "error in (no error)"=w141) -> ("Modbus master out"=w137:refnum<class "Modbus Master.lvclass">, "FV Output"=w131:bool[], "seconds since 1Jan1904 out"=w134:timestamp, "Toggle Output"=w130:bool, "error out"=w140:errorcluster)  [unwired: 4 in, 1 out]
        "FV Output" <- w131
        n24 = disable-structure shown="Enabled" {
          disable-tunnel: w132 -> [w157 _]
          disable-tunnel: [w155 "Loop Rate"] -> w146
          disable-tunnel: [w154 w159] -> w143
          disable-tunnel: w142 -> [w153 _]
          disable-tunnel: w140 -> [w150 w159]
          frame Disabled {
            n25 = call "Modbus Check Sequence Status.vi"("Input Registers"=w153) -> ("Test chamber is in sequence - LDO"=w151:bool, "Test chamber is in sequence - FVIR"=w152:bool)  [unwired: 9 in]
            n26 = call "Modbus Search For Message.vi"("Test chamber is in sequence - LDO"=w151, "Test chamber is in sequence - FVIR"=w152, "error in (no error)"=w150, "Message"="Life Bit", "Modbus Input"=w157) -> ("error out"=w154:errorcluster, "Loop Rate"=w155:u32)  [unwired: 4 in, 1 out]
          }
          frame Enabled {
          }
        }
        n27 = call-poly "Enqueue Message.vi"("error in (no error)"=w143, "Message Data"=w142, "Message"="DisplayValuesFromPLC", "Message Queue"=w139) -> ("error out"=w129:errorcluster)  [unwired: 6 in, 1 out]
      }
      frame "Life Bit" {
        # "No longer used. Delete after a few tests"
        n28 = disable-structure shown="Disabled" {
          disable-tunnel: w172 -> [w192 _]
          disable-tunnel: [w190 u32 400 ("Loop Rate")] -> w171
          disable-tunnel: w170 -> [w186 w195]
          disable-tunnel: w169 -> [w185 w197]
          disable-tunnel: [w184 w195] -> w168
          disable-tunnel: [w183 w197] -> w167
          disable-tunnel: w166 -> [w182 w196]
          disable-tunnel: w165 -> [w181 w198]
          disable-tunnel: w164 -> [w179 w193]
          disable-tunnel: [w178 w193] -> w163
          disable-tunnel: [w177 w196] -> w162
          disable-tunnel: w161 -> [w176 _]
          disable-tunnel: [w175 w198] -> w160
          frame Disabled {
            # "Life Bit"
            n29 = call "Modbus Life Bit Toggle.vi"("FVIR Boolean Array Input"=w182, "Modbus master in"=w179, "UI"=w176, "seconds since 1Jan1904 in"=w185, "Toggle Input"=w186, "error in (no error)"=w181) -> ("Modbus master out"=w178:refnum<class "Modbus Master.lvclass">, "FV Output"=w177:bool[], "seconds since 1Jan1904 out"=w183:timestamp, "Toggle Output"=w184:bool, "error out"=w180:errorcluster)  [unwired: 4 in, 1 out]
            n30 = local read "Input Registers"() -> (w189:u16[])
            n31 = call "Modbus Check Sequence Status.vi"("Input Registers"=w189) -> ("Test chamber is in sequence - LDO"=w187:bool, "Test chamber is in sequence - FVIR"=w188:bool)  [unwired: 9 in]
            n32 = call "Modbus Search For Message.vi"("Test chamber is in sequence - LDO"=w187, "Test chamber is in sequence - FVIR"=w188, "error in (no error)"=w180, "Message"="Read data from PLC", "Modbus Input"=w192) -> ("error out"=w175:errorcluster, "Loop Rate"=w190:u32)  [unwired: 4 in, 1 out]
          }
          frame Enabled {
          }
        }
      }
      frame "Write bit pattern to FVIR and LDO" {
        # "LDO register 40034"
        # "LDO register 40011"
        # "FVIR register 40001"
        # "Here the toggle bit is used for writing the value at address 0. Afterwards\nit is inverted and pass through, so next time the lifebit will be toggled."
        n33 = Boolean Array To Number(Boolean array=w205) -> (number=w221:u32)
        n34 = call-dynamic "Write Single Holding Register.vi"("error in"=w216, "register to write"=w221, "address"=u16 0 ("starting address"), "Modbus master in"=w223) -> ("error out"=w219:errorcluster, "Modbus master out"=w220:refnum<class "Modbus Master.lvclass">)  [unwired: 6 in]
        n35 = Boolean Array To Number(Boolean array=w207) -> (number=→"LDO Output Value":u32)
        n36 = Boolean Array To Number(Boolean array=w207) -> (number=w217:u32)
        n37 = call-dynamic "Write Single Holding Register.vi"("error in"=w219, "register to write"=w217, "address"=u16 10, "Modbus master in"=w220) -> ("error out"=w215:errorcluster, "Modbus master out"=w213:refnum<class "Modbus Master.lvclass">)  [unwired: 6 in]
        n38 = Boolean Array To Number(Boolean array=w209) -> (number=w210:u32)
        n39 = call-dynamic "Write Single Holding Register.vi"("error in"=w215, "register to write"=w210, "address"=u16 33, "Modbus master in"=w213) -> ("error out"=w214:errorcluster, "Modbus master out"=w212:refnum<class "Modbus Master.lvclass">)  [unwired: 6 in]
        n40 = call-poly "Enqueue Message.vi"("Priority Message? (F)"=TRUE, "error in (no error)"=w214, "Message"="Read data from PLC", "Message Queue"=w201) -> ("error out"=w202:errorcluster)  [unwired: 6 in, 1 out]
        "LDO Array 1" <- w207
        "LDO Array 2" <- w209
      }
      frame "Reset all button signals to PLC" {
        # "Reset all the buttons signals after watchdog pause."
        n41 = call-dynamic "Write Multiple Holding Registers.vi"("error in"=w235, "registers to write"=u16[] [99, 99, 99, 99, 99, 99, 99, 99, 99, 99, 99, 99], "starting address"=u16 10, "Modbus master in"=w233) -> ("error out"=w231:errorcluster, "Modbus master out"=w234:refnum<class "Modbus Master.lvclass">)  [unwired: 6 in]
      }
      frame "Exit" {
        # "Flushing the WD helper loop in order to quick close down, if the operator is pressing Exit"
        # "When main loop receive \"Exit\" on its queue, the exit case will commit \"Exit\" to its helper loop"
        # "Stop the VI"
        n42 = Flush Queue(queue=w246, error in (no error)=w247) -> (queue out=w245:refnum<queue>, error out=w244:errorcluster)  [unwired: 1 out]
        n43 = call-dynamic "Shutdown.vi"("error in"=w244, "Modbus master in"=w243) -> ("error out"=w248:errorcluster)  [unwired: 9 in]
        n44 = call <vilib>:"Clear Errors.vi"("error in (no error)"=w248) -> ("error out"=w242:errorcluster)  [unwired: 5 in, 1 out]
        n45 = case shown="Error" w242 {
          selector: w242 -> [w265 w268]
          tunnel: w237 -> [w257 w266]
          tunnel: [w263 w267] -> w241
          frame No Error {
            n46 = call-poly "Enqueue Message.vi"("error in (no error)"=w265, "Message Data"="Succesfully disconnected with Modbus TCP/IP..." ("Acquiring and Logging..."), "Message"="Update Status - FVIR", "Message Queue"=w257) -> ("error out"=w264:errorcluster, "dup Message Queue"=w262:refnum<queue>)  [unwired: 6 in]
            n47 = call-poly "Enqueue Message.vi"("error in (no error)"=w264, "Message Data"="Succesfully disconnected with Modbus TCP/IP..." ("Acquiring and Logging..."), "Message"="Update Status - LDO", "Message Queue"=w262) -> ("error out"=w263:errorcluster)  [unwired: 6 in, 1 out]
          }
          frame Error {
            n48 = call-poly "Enqueue Message.vi"("error in (no error)"=w268, "Message Data"="Error with disconnecting with Modbus TCP/IP..." ("Acquiring and Logging..."), "Message"="Update Status - FVIR", "Message Queue"=w266) -> ("error out"=w274:errorcluster, "dup Message Queue"=w273:refnum<queue>)  [unwired: 6 in]
            n49 = call-poly "Enqueue Message.vi"("error in (no error)"=w274, "Message Data"="Error with disconnecting with Modbus TCP/IP..." ("Acquiring and Logging..."), "Message"="Update Status - LDO", "Message Queue"=w273) -> ("error out"=w267:errorcluster)  [unwired: 6 in, 1 out]
          }
        }
        n50 = call-poly "Enqueue Message.vi"("Priority Message? (F)"=TRUE, "error in (no error)"=w241, "Message"="Exit", "Message Queue"=w245) -> ("error out"=w253:errorcluster, "dup Message Queue"=w236:refnum<queue>)  [unwired: 6 in]
        n51 = Release Queue(queue=w236, error in (no error)=w253) -> (error out=w240:errorcluster)  [unwired: 1 in, 2 out]
      }
      frame "---- LDO Test ----" {
      }
      frame "StartTestCaseLDO" {
        n52 = Replace Array Subset(array=w290, new element=TRUE ("new element/subarray"), index=2) -> (w289:bool[])
        n53 = call-poly "Enqueue Message.vi"("Priority Message? (F)"=TRUE, "error in (no error)"=w293, "Message"="Write bit pattern to FVIR and LDO", "Message Queue"=w297) -> ("error out"=w296:errorcluster)  [unwired: 6 in, 1 out]
      }
      frame "StopTestCaseLDO" {
        n54 = Replace Array Subset(array=w305, new element=FALSE ("new element/subarray"), index=2) -> (w304:bool[])
        n55 = call-poly "Enqueue Message.vi"("error in (no error)"=w308, "Message"="ResetTestLDO", "Message Queue"=w298) -> ("error out"=w307:errorcluster)  [unwired: 7 in, 1 out]
        n56 = call-poly "Enqueue Message.vi"("Priority Message? (F)"=TRUE, "error in (no error)"=w307, "Message"="Write bit pattern to FVIR and LDO", "Message Queue"=w298) -> ("error out"=w310:errorcluster)  [unwired: 6 in, 1 out]
      }
      frame "ResetTestLDO" {
        # "Writing to PLC with value 0 at address 10. This will reset the LDO test in the PLC"
        n57 = call-dynamic "Write Single Holding Register.vi"("error in"=w330, "register to write"=u16 0, "address"=u16 10 ("starting address"), "Modbus master in"=w328) -> ("error out"=w324:errorcluster, "Modbus master out"=w329:refnum<class "Modbus Master.lvclass">)  [unwired: 6 in]
        n58 = call-poly "Enqueue Message.vi"("Priority Message? (F)"=TRUE, "error in (no error)"=w324, "Message"="Write bit pattern to FVIR and LDO", "Message Queue"=w325) -> ("error out"=w322:errorcluster)  [unwired: 6 in, 1 out]
      }
      frame "SendParamToPLCLDO" {
        # "This for loop basically just takes the array from the Modbus queue and write\neach index value to each unique register. I.e. the first control value from the HMI\nwhich is \"Time delay of change direction of mannequin actuators\" is written to \nregister 1 (40002). The next control value from the HMI is the \"Number of\nmannequin movement\" and that value is written to register 2 (40003). \nThis continues until there are no further values in the array.\n\n(Register 0 is the bit combination from, regsiter 40001). See\nthe case  \"Writing to register 40001)"
        n59 = Variant To Data(type=i32[] [], Variant=w345) -> (data=w342:i32[], error out=w339:errorcluster)  [unwired: 1 in]
        n60 = call "Modbus Send Parameters LDO.vi"("error in (no error)"=w339, "Array in"=w342, "Modbus Master in"=w341) -> ("error out"=w338:errorcluster, "Modbus Master out"=w340:refnum<class "Modbus Master.lvclass">)  [unwired: 7 in]
        n61 = call-poly "Enqueue Message.vi"("Priority Message? (F)"=TRUE, "error in (no error)"=w338, "Message"="Write bit pattern to FVIR and LDO", "Message Queue"=w347) -> ("error out"=w343:errorcluster)  [unwired: 6 in, 1 out]
      }
      frame "TimeoutRequestGetDataLDO" {
        # "#What is this doing?"
        n62 = disable-structure shown="Disabled" {
          disable-tunnel: w358 -> [w367 w369]
          disable-tunnel: [w365 w369] -> w357
          disable-tunnel: w355 -> [w364 w370]
          disable-tunnel: [w362 w370] -> w353
          disable-tunnel: w352 -> [w361 _]
          frame Disabled {
            # "For LDO data only, the required registers goes from 31 to 56."
            n63 = call-dynamic "Read Input Registers.vi"("error in"=w364, "number of inputs"=u16 56, "starting address"=u16 31, "Modbus master in"=w367) -> ("error out"=w363:errorcluster, "register values"=w360:u16[], "Modbus master out"=w365:refnum<class "Modbus Master.lvclass">)  [unwired: 5 in]
            n64 = call-poly "Enqueue Message.vi"("error in (no error)"=w363, "Message Data"=w360, "Message"="CheckBeforeWriteDataLDO", "Message Queue"=w361) -> ("error out"=w362:errorcluster)  [unwired: 6 in, 1 out]
          }
          frame Enabled {
          }
        }
      }
      frame "WaterOutletOpenLDO" {
        n65 = Replace Array Subset(array=w378, new element=TRUE ("new element/subarray"), index=3) -> (w377:bool[])
        n66 = call-poly "Enqueue Message.vi"("Priority Message? (F)"=TRUE, "error in (no error)"=w381, "Message"="Write bit pattern to FVIR and LDO", "Message Queue"=w385) -> ("error out"=w384:errorcluster)  [unwired: 6 in, 1 out]
      }
      frame "WaterOutletCloseLDO" {
        n67 = Replace Array Subset(array=w393, new element=FALSE ("new element/subarray"), index=3) -> (w392:bool[])
        n68 = call-poly "Enqueue Message.vi"("Priority Message? (F)"=TRUE, "error in (no error)"=w396, "Message"="Write bit pattern to FVIR and LDO", "Message Queue"=w400) -> ("error out"=w399:errorcluster)  [unwired: 6 in, 1 out]
      }
      frame "WaterInletOpenLDO" {
        n69 = Replace Array Subset(array=w408, new element=TRUE ("new element/subarray"), index=4) -> (w407:bool[])
        n70 = call-poly "Enqueue Message.vi"("Priority Message? (F)"=TRUE, "error in (no error)"=w411, "Message"="Write bit pattern to FVIR and LDO", "Message Queue"=w415) -> ("error out"=w414:errorcluster)  [unwired: 6 in, 1 out]
      }
      frame "WaterInletCloseLDO" {
        n71 = Replace Array Subset(array=w423, new element=FALSE ("new element/subarray"), index=4) -> (w422:bool[])
        n72 = call-poly "Enqueue Message.vi"("Priority Message? (F)"=TRUE, "error in (no error)"=w426, "Message"="Write bit pattern to FVIR and LDO", "Message Queue"=w430) -> ("error out"=w429:errorcluster)  [unwired: 6 in, 1 out]
      }
      frame "GasSolenoidOpenLDO" {
        n73 = Replace Array Subset(array=w438, new element=TRUE ("new element/subarray"), index=5) -> (w437:bool[])
        n74 = call-poly "Enqueue Message.vi"("Priority Message? (F)"=TRUE, "error in (no error)"=w441, "Message"="Write bit pattern to FVIR and LDO", "Message Queue"=w445) -> ("error out"=w444:errorcluster)  [unwired: 6 in, 1 out]
      }
      frame "GasSolenoidCloseLDO" {
        n75 = Replace Array Subset(array=w453, new element=FALSE ("new element/subarray"), index=5) -> (w452:bool[])
        n76 = call-poly "Enqueue Message.vi"("Priority Message? (F)"=TRUE, "error in (no error)"=w456, "Message"="Write bit pattern to FVIR and LDO", "Message Queue"=w460) -> ("error out"=w459:errorcluster)  [unwired: 6 in, 1 out]
      }
      frame "WaterFlowStartLDO" {
        n77 = Replace Array Subset(array=w468, new element=TRUE ("new element/subarray"), index=6) -> (w467:bool[])
        n78 = call-poly "Enqueue Message.vi"("Priority Message? (F)"=TRUE, "error in (no error)"=w471, "Message"="Write bit pattern to FVIR and LDO", "Message Queue"=w475) -> ("error out"=w474:errorcluster)  [unwired: 6 in, 1 out]
      }
      frame "WaterFlowStartZeroLDO" {
        n79 = Replace Array Subset(array=w483, new element=FALSE ("new element/subarray"), index=6) -> (w482:bool[])
        n80 = call-poly "Enqueue Message.vi"("Priority Message? (F)"=TRUE, "error in (no error)"=w486, "Message"="Write bit pattern to FVIR and LDO", "Message Queue"=w490) -> ("error out"=w489:errorcluster)  [unwired: 6 in, 1 out]
      }
      frame "WaterFlowStopLDO" {
        n81 = Replace Array Subset(array=w496, new element=TRUE ("new element/subarray"), index=8) -> (w495:bool[])
        n82 = call-poly "Enqueue Message.vi"("Priority Message? (F)"=TRUE, "error in (no error)"=w497, "Message"="Write bit pattern to FVIR and LDO", "Message Queue"=w498) -> ("error out"=w494:errorcluster)  [unwired: 6 in, 1 out]
      }
      frame "WaterFlowStopZeroLDO" {
        n83 = Replace Array Subset(array=w513, new element=FALSE ("new element/subarray"), index=8) -> (w512:bool[])
        n84 = call-poly "Enqueue Message.vi"("Priority Message? (F)"=TRUE, "error in (no error)"=w510, "Message"="Write bit pattern to FVIR and LDO", "Message Queue"=w511) -> ("error out"=w509:errorcluster)  [unwired: 6 in, 1 out]
      }
      frame "TempChangeDRK375_LDO" {
        # "Write the temperature to the PLC"
        n85 = Variant To Data(error in=w536, type=0.0 ("Numeric"), Variant=w535) -> (data=w530:dbl, error out=w531:errorcluster)
        n86 = call "UTILITY Modbus 32bit Number to 16bit Array.vi"("error in"=w531, "32-bit IEEE 754"=w530) -> ("error out"=w534:errorcluster, "U16 Array Representation"=w532:u16[])  [unwired: 8 in]
        n87 = call-dynamic "Write Multiple Holding Registers.vi"("error in"=w534, "registers to write"=w532, "starting address"=u16 13 ("address"), "Modbus master in"=w529) -> ("error out"=w525:errorcluster, "Modbus master out"=w528:refnum<class "Modbus Master.lvclass">)  [unwired: 6 in]
        n88 = call-poly "Enqueue Message.vi"("Priority Message? (F)"=TRUE, "error in (no error)"=w525, "Message"="Write bit pattern to FVIR and LDO", "Message Queue"=w526) -> ("error out"=w524:errorcluster)  [unwired: 6 in, 1 out]
      }
      frame "ValveChangeDRK375_LDO" {
        # "Write the Valve position to the PLC"
        n89 = Variant To Data(error in=w557, type=0.0 ("Numeric"), Variant=w556) -> (data=w554:dbl, error out=w555:errorcluster)
        n90 = call "UTILITY Modbus 32bit Number to 16bit Array.vi"("error in"=w555, "32-bit IEEE 754"=w554) -> ("error out"=w545:errorcluster, "U16 Array Representation"=w544:u16[])  [unwired: 8 in]
        n91 = call-dynamic "Write Multiple Holding Registers.vi"("error in"=w545, "registers to write"=w544, "starting address"=u16 15 ("address"), "Modbus master in"=w553) -> ("error out"=w542:errorcluster, "Modbus master out"=w552:refnum<class "Modbus Master.lvclass">)  [unwired: 6 in]
        n92 = call-poly "Enqueue Message.vi"("Priority Message? (F)"=TRUE, "error in (no error)"=w542, "Message"="Write bit pattern to FVIR and LDO", "Message Queue"=w550) -> ("error out"=w549:errorcluster)  [unwired: 6 in, 1 out]
      }
      frame "ValveChangeEPV_LDO" {
        n93 = Variant To Data(error in=w578, type=0.0 ("Numeric"), Variant=w577) -> (data=w575:dbl, error out=w576:errorcluster)
        n94 = call "UTILITY Modbus 32bit Number to 16bit Array.vi"("error in"=w576, "32-bit IEEE 754"=w575) -> ("error out"=w574:errorcluster, "U16 Array Representation"=w572:u16[])  [unwired: 8 in]
        n95 = call-dynamic "Write Multiple Holding Registers.vi"("error in"=w574, "registers to write"=w572, "starting address"=u16 11 ("address"), "Modbus master in"=w571) -> ("error out"=w568:errorcluster, "Modbus master out"=w570:refnum<class "Modbus Master.lvclass">)  [unwired: 6 in]
        n96 = call-poly "Enqueue Message.vi"("Priority Message? (F)"=TRUE, "error in (no error)"=w568, "Message"="Write bit pattern to FVIR and LDO", "Message Queue"=w566) -> ("error out"=w567:errorcluster)  [unwired: 6 in, 1 out]
      }
      frame "Output_Flow_Target_LDO" {
        n97 = Variant To Data(error in=w594, type=0.0 ("Numeric"), Variant=w593) -> (data=w597:dbl, error out=w598:errorcluster)
        n98 = call "UTILITY Modbus 32bit Number to 16bit Array.vi"("error in"=w598, "32-bit IEEE 754"=w597) -> ("error out"=w600:errorcluster, "U16 Array Representation"=w599:u16[])  [unwired: 8 in]
        n99 = call-dynamic "Write Multiple Holding Registers.vi"("error in"=w600, "registers to write"=w599, "starting address"=u16 31 ("address"), "Modbus master in"=w592) -> ("error out"=w589:errorcluster, "Modbus master out"=w591:refnum<class "Modbus Master.lvclass">)  [unwired: 6 in]
        n100 = call-poly "Enqueue Message.vi"("Priority Message? (F)"=TRUE, "error in (no error)"=w589, "Message"="Write bit pattern to FVIR and LDO", "Message Queue"=w587) -> ("error out"=w588:errorcluster)  [unwired: 6 in, 1 out]
      }
      frame "OilSpray08Open" {
        n101 = Replace Array Subset(array=w612, new element=TRUE ("new element/subarray"), index=9) -> (w611:bool[])
        n102 = call-poly "Enqueue Message.vi"("Priority Message? (F)"=TRUE, "error in (no error)"=w615, "Message"="Write bit pattern to FVIR and LDO", "Message Queue"=w619) -> ("error out"=w618:errorcluster)  [unwired: 6 in, 1 out]
      }
      frame "OilSpray08Close" {
        n103 = Replace Array Subset(array=w627, new element=FALSE ("new element/subarray"), index=9) -> (w626:bool[])
        n104 = call-poly "Enqueue Message.vi"("Priority Message? (F)"=TRUE, "error in (no error)"=w630, "Message"="Write bit pattern to FVIR and LDO", "Message Queue"=w634) -> ("error out"=w633:errorcluster)  [unwired: 6 in, 1 out]
      }
      frame "OilSpray11Open" {
        n105 = Replace Array Subset(array=w642, new element=TRUE ("new element/subarray"), index=10) -> (w641:bool[])
        n106 = call-poly "Enqueue Message.vi"("Priority Message? (F)"=TRUE, "error in (no error)"=w645, "Message"="Write bit pattern to FVIR and LDO", "Message Queue"=w649) -> ("error out"=w648:errorcluster)  [unwired: 6 in, 1 out]
      }
      frame "OilSpray11Close" {
        n107 = Replace Array Subset(array=w657, new element=FALSE ("new element/subarray"), index=10) -> (w656:bool[])
        n108 = call-poly "Enqueue Message.vi"("Priority Message? (F)"=TRUE, "error in (no error)"=w660, "Message"="Write bit pattern to FVIR and LDO", "Message Queue"=w664) -> ("error out"=w663:errorcluster)  [unwired: 6 in, 1 out]
      }
      frame "OilSpray133Open" {
        n109 = Replace Array Subset(array=w672, new element=TRUE ("new element/subarray"), index=11) -> (w671:bool[])
        n110 = call-poly "Enqueue Message.vi"("Priority Message? (F)"=TRUE, "error in (no error)"=w675, "Message"="Write bit pattern to FVIR and LDO", "Message Queue"=w679) -> ("error out"=w678:errorcluster)  [unwired: 6 in, 1 out]
      }
      frame "OilSpray133Close" {
        n111 = Replace Array Subset(array=w687, new element=FALSE ("new element/subarray"), index=11) -> (w686:bool[])
        n112 = call-poly "Enqueue Message.vi"("Priority Message? (F)"=TRUE, "error in (no error)"=w690, "Message"="Write bit pattern to FVIR and LDO", "Message Queue"=w694) -> ("error out"=w693:errorcluster)  [unwired: 6 in, 1 out]
      }
      frame "HeaterON_LDO" {
        n113 = Replace Array Subset(array=w702, new element=TRUE ("new element/subarray"), index=12) -> (w701:bool[])
        n114 = call-poly "Enqueue Message.vi"("Priority Message? (F)"=TRUE, "error in (no error)"=w705, "Message"="Write bit pattern to FVIR and LDO", "Message Queue"=w709) -> ("error out"=w708:errorcluster)  [unwired: 6 in, 1 out]
      }
      frame "HeaterOFF_LDO" {
        n115 = Replace Array Subset(array=w717, new element=FALSE ("new element/subarray"), index=12) -> (w716:bool[])
        n116 = call-poly "Enqueue Message.vi"("Priority Message? (F)"=TRUE, "error in (no error)"=w720, "Message"="Write bit pattern to FVIR and LDO", "Message Queue"=w724) -> ("error out"=w723:errorcluster)  [unwired: 6 in, 1 out]
      }
      frame "ResetFlowMeter_ON_LDO" {
        n117 = Replace Array Subset(array=w736, new element=TRUE ("new element/subarray"), index=13) -> (w735:bool[])
        n118 = call-poly "Enqueue Message.vi"("Priority Message? (F)"=TRUE, "error in (no error)"=w733, "Message"="Write bit pattern to FVIR and LDO", "Message Queue"=w734) -> ("error out"=w732:errorcluster)  [unwired: 6 in, 1 out]
      }
      frame "ResetFlowMeter_OFF_LDO" {
        n119 = Replace Array Subset(array=w751, new element=FALSE ("new element/subarray"), index=13) -> (w750:bool[])
        n120 = call-poly "Enqueue Message.vi"("Priority Message? (F)"=TRUE, "error in (no error)"=w748, "Message"="Write bit pattern to FVIR and LDO", "Message Queue"=w749) -> ("error out"=w747:errorcluster)  [unwired: 6 in, 1 out]
      }
      frame "Water_Heater_Status_ON_LDO" {
        n121 = Replace Array Subset(array=w764, new element=TRUE ("new element/subarray"), index=14) -> (w763:bool[])
        n122 = call-poly "Enqueue Message.vi"("Priority Message? (F)"=TRUE, "error in (no error)"=w760, "Message"="Write bit pattern to FVIR and LDO", "Message Queue"=w761) -> ("error out"=w759:errorcluster)  [unwired: 6 in, 1 out]
      }
      frame "Water_Heater_Status_OFF_LDO" {
        n123 = Replace Array Subset(array=w779, new element=FALSE ("new element/subarray"), index=14) -> (w778:bool[])
        n124 = call-poly "Enqueue Message.vi"("Priority Message? (F)"=TRUE, "error in (no error)"=w775, "Message"="Write bit pattern to FVIR and LDO", "Message Queue"=w776) -> ("error out"=w774:errorcluster)  [unwired: 6 in, 1 out]
      }
      frame "PID_Selector_OFF_LDO" {
        n125 = Replace Array Subset(array=w794, new element=FALSE ("new element/subarray"), index=15) -> (w793:bool[])
        n126 = call-poly "Enqueue Message.vi"("Priority Message? (F)"=TRUE, "error in (no error)"=w790, "Message"="Write bit pattern to FVIR and LDO", "Message Queue"=w791) -> ("error out"=w789:errorcluster)  [unwired: 6 in, 1 out]
      }
      frame "ConveyorON" {
        n127 = call-poly "Enqueue Message.vi"("Priority Message? (F)"=TRUE, "error in (no error)"=w806, "Message"="Write bit pattern to FVIR and LDO", "Message Queue"=w805) -> ("error out"=w807:errorcluster)  [unwired: 6 in, 1 out]
        n128 = Replace Array Subset(array=w804, new element=TRUE ("new element/subarray"), index=0) -> (w803:bool[])
      }
      frame "ConveyorOFF" {
        n129 = call-poly "Enqueue Message.vi"("Priority Message? (F)"=TRUE, "error in (no error)"=w820, "Message"="Write bit pattern to FVIR and LDO", "Message Queue"=w821) -> ("error out"=w822:errorcluster)  [unwired: 6 in, 1 out]
        n130 = Replace Array Subset(array=w818, new element=FALSE ("new element/subarray"), index=0) -> (w819:bool[])
      }
      frame "BlowerON" {
        n131 = call-poly "Enqueue Message.vi"("Priority Message? (F)"=TRUE, "error in (no error)"=w836, "Message"="Write bit pattern to FVIR and LDO", "Message Queue"=w835) -> ("error out"=w837:errorcluster)  [unwired: 6 in, 1 out]
        n132 = Replace Array Subset(array=w834, new element=TRUE ("new element/subarray"), index=7) -> (w833:bool[])
      }
      frame "BlowerOFF" {
        n133 = Replace Array Subset(array=w849, new element=FALSE ("new element/subarray"), index=7) -> (w848:bool[])
        n134 = call-poly "Enqueue Message.vi"("Priority Message? (F)"=TRUE, "error in (no error)"=w851, "Message"="Write bit pattern to FVIR and LDO", "Message Queue"=w850) -> ("error out"=w852:errorcluster)  [unwired: 6 in, 1 out]
      }
      frame "---- FVIR Test ----" {
      }
      frame "StartTestCaseFVIR" {
        # "FIX from here and the rest. Instead of using old Watchdog loop, then just queue to Modbus to write again status back to PLC"
        n135 = Replace Array Subset(array=w877, new element=TRUE ("new element/subarray"), index=1) -> (w876:bool[])
        n136 = call-poly "Enqueue Message.vi"("Priority Message? (F)"=TRUE, "error in (no error)"=w879, "Message"="Write bit pattern to FVIR and LDO", "Message Queue"=w882) -> ("error out"=w881:errorcluster)  [unwired: 6 in, 1 out]
      }
      frame "StopTestCaseFVIR" {
        n137 = Replace Array Subset(array=w895, new element=FALSE ("new element/subarray"), index=1) -> (w894:bool[])
        n138 = call-poly "Enqueue Message.vi"("Priority Message? (F)"=TRUE, "error in (no error)"=w891, "Message"="ResetTestFVIR", "Message Queue"=w883) -> ("error out"=w886:errorcluster)  [unwired: 6 in, 1 out]
      }
      frame "ResetTestFVIR" {
        # "Writing to PLC with value 0 at address 7"
        n139 = call-dynamic "Write Single Holding Register.vi"("error in"=w913, "register to write"=u16 0, "address"=u16 7 ("starting address"), "Modbus master in"=w911) -> ("error out"=w907:errorcluster, "Modbus master out"=w912:refnum<class "Modbus Master.lvclass">)  [unwired: 6 in]
        n140 = call-poly "Enqueue Message.vi"("Priority Message? (F)"=TRUE, "error in (no error)"=w907, "Message"="Write bit pattern to FVIR and LDO", "Message Queue"=w908) -> ("error out"=w905:errorcluster)  [unwired: 6 in, 1 out]
      }
      frame "SendParamToPLCFVIR" {
        n141 = Variant To Data(type=i32[] [], Variant=w928) -> (data=w925:i32[], error out=w922:errorcluster)  [unwired: 1 in]
        n142 = call "Modbus Send Parameters FVIR.vi"("error in (no error)"=w922, "Array"=w925, "Modbus Master in"=w924) -> ("error out"=w921:errorcluster, "Modbus Master out"=w923:refnum<class "Modbus Master.lvclass">)  [unwired: 7 in]
        n143 = call-poly "Enqueue Message.vi"("Priority Message? (F)"=TRUE, "error in (no error)"=w921, "Message"="Write bit pattern to FVIR and LDO", "Message Queue"=w930) -> ("error out"=w926:errorcluster)  [unwired: 6 in, 1 out]
      }
      frame "TimeoutRequestGetDataFVIR" {
        # "#What is this doing? For FVIR data only, the required registers goes from 0 to 30."
        n144 = disable-structure shown="Disabled" {
          disable-tunnel: w942 -> [w956 w959]
          disable-tunnel: [w954 w959] -> w941
          disable-tunnel: [w952 w958] -> w938
          disable-tunnel: w937 -> [w951 _]
          disable-tunnel: w936 -> [w949 w958]
          disable-tunnel: w935 -> [w946 _]
          frame Disabled {
            n145 = Variant To Data(error in=w949, type=i32[] [], Variant=w946) -> (data=w944:i32[], error out=w948:errorcluster)
            n146 = call-dynamic "Read Input Registers.vi"("error in"=w948, "number of inputs"=u16 30, "starting address"=u16 0, "Modbus master in"=w956) -> ("error out"=w953:errorcluster, "register values"=w945:u16[], "Modbus master out"=w954:refnum<class "Modbus Master.lvclass">)  [unwired: 5 in]
            n147 = Build Array (concatenate)(w945, w944) -> (w943:i32[])
            n148 = call-poly "Enqueue Message.vi"("error in (no error)"=w953, "Message Data"=w943, "Message"="CheckBeforeWriteDataFVIR", "Message Queue"=w951) -> ("error out"=w952:errorcluster)  [unwired: 6 in, 1 out]
          }
          frame Enabled {
          }
        }
      }
      frame "StartManSeq" {
        n149 = Replace Array Subset(array=w968, new element=TRUE ("new element/subarray"), index=2) -> (w967:bool[])
        n150 = call-poly "Enqueue Message.vi"("Priority Message? (F)"=TRUE, "error in (no error)"=w970, "Message"="Write bit pattern to FVIR and LDO", "Message Queue"=w974) -> ("error out"=w973:errorcluster)  [unwired: 6 in, 1 out]
      }
      frame "StopManSeq" {
        n151 = Replace Array Subset(array=w983, new element=FALSE ("new element/subarray"), index=2) -> (w982:bool[])
        n152 = call-poly "Enqueue Message.vi"("Priority Message? (F)"=TRUE, "error in (no error)"=w985, "Message"="Write bit pattern to FVIR and LDO", "Message Queue"=w989) -> ("error out"=w988:errorcluster)  [unwired: 6 in, 1 out]
      }
      frame "WaterOutletOpenFVIR" {
        n153 = Replace Array Subset(array=w998, new element=TRUE ("new element/subarray"), index=3) -> (w997:bool[])
        n154 = call-poly "Enqueue Message.vi"("Priority Message? (F)"=TRUE, "error in (no error)"=w1000, "Message"="Write bit pattern to FVIR and LDO", "Message Queue"=w1004) -> ("error out"=w1003:errorcluster)  [unwired: 6 in, 1 out]
      }
      frame "WaterOutletCloseFVIR" {
        n155 = Replace Array Subset(array=w1013, new element=FALSE ("new element/subarray"), index=3) -> (w1012:bool[])
        n156 = call-poly "Enqueue Message.vi"("Priority Message? (F)"=TRUE, "error in (no error)"=w1015, "Message"="Write bit pattern to FVIR and LDO", "Message Queue"=w1019) -> ("error out"=w1018:errorcluster)  [unwired: 6 in, 1 out]
      }
      frame "WaterInletOpenFVIR" {
        n157 = Replace Array Subset(array=w1028, new element=TRUE ("new element/subarray"), index=4) -> (w1027:bool[])
        n158 = call-poly "Enqueue Message.vi"("Priority Message? (F)"=TRUE, "error in (no error)"=w1030, "Message"="Write bit pattern to FVIR and LDO", "Message Queue"=w1034) -> ("error out"=w1033:errorcluster)  [unwired: 6 in, 1 out]
      }
      frame "WaterInletCloseFVIR" {
        n159 = Replace Array Subset(array=w1043, new element=FALSE ("new element/subarray"), index=4) -> (w1042:bool[])
        n160 = call-poly "Enqueue Message.vi"("Priority Message? (F)"=TRUE, "error in (no error)"=w1045, "Message"="Write bit pattern to FVIR and LDO", "Message Queue"=w1049) -> ("error out"=w1048:errorcluster)  [unwired: 6 in, 1 out]
      }
      frame "GasSolenoidOpenFVIR" {
        n161 = Replace Array Subset(array=w1058, new element=TRUE ("new element/subarray"), index=5) -> (w1057:bool[])
        n162 = call-poly "Enqueue Message.vi"("Priority Message? (F)"=TRUE, "error in (no error)"=w1060, "Message"="Write bit pattern to FVIR and LDO", "Message Queue"=w1064) -> ("error out"=w1063:errorcluster)  [unwired: 6 in, 1 out]
      }
      frame "GasSolenoidCloseFVIR" {
        n163 = Replace Array Subset(array=w1073, new element=FALSE ("new element/subarray"), index=5) -> (w1072:bool[])
        n164 = call-poly "Enqueue Message.vi"("Priority Message? (F)"=TRUE, "error in (no error)"=w1075, "Message"="Write bit pattern to FVIR and LDO", "Message Queue"=w1079) -> ("error out"=w1078:errorcluster)  [unwired: 6 in, 1 out]
      }
      frame "WaterFlowStartFVIR" {
        n165 = Replace Array Subset(array=w1088, new element=TRUE ("new element/subarray"), index=6) -> (w1087:bool[])
        n166 = call-poly "Enqueue Message.vi"("Priority Message? (F)"=TRUE, "error in (no error)"=w1090, "Message"="Write bit pattern to FVIR and LDO", "Message Queue"=w1094) -> ("error out"=w1093:errorcluster)  [unwired: 6 in, 1 out]
      }
      frame "WaterFlowStartZeroFVIR" {
        n167 = Replace Array Subset(array=w1103, new element=FALSE ("new element/subarray"), index=6) -> (w1102:bool[])
        n168 = call-poly "Enqueue Message.vi"("Priority Message? (F)"=TRUE, "error in (no error)"=w1105, "Message"="Write bit pattern to FVIR and LDO", "Message Queue"=w1109) -> ("error out"=w1108:errorcluster)  [unwired: 6 in, 1 out]
      }
      frame "WaterFlowStopFVIR" {
        n169 = Replace Array Subset(array=w1118, new element=TRUE ("new element/subarray"), index=8) -> (w1117:bool[])
        n170 = call-poly "Enqueue Message.vi"("Priority Message? (F)"=TRUE, "error in (no error)"=w1120, "Message"="Write bit pattern to FVIR and LDO", "Message Queue"=w1124) -> ("error out"=w1123:errorcluster)  [unwired: 6 in, 1 out]
      }
      frame "WaterFlowStopZeroFVIR" {
        n171 = Replace Array Subset(array=w1133, new element=FALSE ("new element/subarray"), index=8) -> (w1132:bool[])
        n172 = call-poly "Enqueue Message.vi"("Priority Message? (F)"=TRUE, "error in (no error)"=w1135, "Message"="Write bit pattern to FVIR and LDO", "Message Queue"=w1139) -> ("error out"=w1138:errorcluster)  [unwired: 6 in, 1 out]
      }
      frame "TempChangeDRK375_FVIR" {
        # "Write the temperature to the PLC"
        n173 = Variant To Data(error in=w1155, type=0.0 ("Numeric"), Variant=w1154) -> (data=w1149:dbl, error out=w1150:errorcluster)
        n174 = call "UTILITY Modbus 32bit Number to 16bit Array.vi"("error in"=w1150, "32-bit IEEE 754"=w1149) -> ("error out"=w1153:errorcluster, "U16 Array Representation"=w1151:u16[])  [unwired: 8 in]
        n175 = call-dynamic "Write Multiple Holding Registers.vi"("error in"=w1153, "registers to write"=w1151, "starting address"=u16 51 ("address"), "Modbus master in"=w1148) -> ("error out"=w1144:errorcluster, "Modbus master out"=w1147:refnum<class "Modbus Master.lvclass">)  [unwired: 6 in]
        n176 = call-poly "Enqueue Message.vi"("Priority Message? (F)"=TRUE, "error in (no error)"=w1144, "Message"="Write bit pattern to FVIR and LDO", "Message Queue"=w1145) -> ("error out"=w1143:errorcluster)  [unwired: 6 in, 1 out]
      }
      frame "ValveChangeDRK375_FVIR" {
        # "Write the Valve position to the PLC"
        n177 = Variant To Data(error in=w1176, type=0.0 ("Numeric"), Variant=w1175) -> (data=w1170:dbl, error out=w1171:errorcluster)
        n178 = call "UTILITY Modbus 32bit Number to 16bit Array.vi"("error in"=w1171, "32-bit IEEE 754"=w1170) -> ("error out"=w1174:errorcluster, "U16 Array Representation"=w1173:u16[])  [unwired: 8 in]
        n179 = call-dynamic "Write Multiple Holding Registers.vi"("error in"=w1174, "registers to write"=w1173, "starting address"=u16 53 ("address"), "Modbus master in"=w1169) -> ("error out"=w1165:errorcluster, "Modbus master out"=w1168:refnum<class "Modbus Master.lvclass">)  [unwired: 6 in]
        n180 = call-poly "Enqueue Message.vi"("Priority Message? (F)"=TRUE, "error in (no error)"=w1165, "Message"="Write bit pattern to FVIR and LDO", "Message Queue"=w1166) -> ("error out"=w1164:errorcluster)  [unwired: 6 in, 1 out]
      }
      frame "ValveChangeEPV_FVIR" {
        n181 = Variant To Data(error in=w1197, type=0.0 ("Numeric"), Variant=w1196) -> (data=w1194:dbl, error out=w1195:errorcluster)
        n182 = call "UTILITY Modbus 32bit Number to 16bit Array.vi"("error in"=w1195, "32-bit IEEE 754"=w1194) -> ("error out"=w1193:errorcluster, "U16 Array Representation"=w1191:u16[])  [unwired: 8 in]
        n183 = call-dynamic "Write Multiple Holding Registers.vi"("error in"=w1193, "registers to write"=w1191, "starting address"=u16 49 ("address"), "Modbus master in"=w1190) -> ("error out"=w1187:errorcluster, "Modbus master out"=w1189:refnum<class "Modbus Master.lvclass">)  [unwired: 6 in]
        n184 = call-poly "Enqueue Message.vi"("Priority Message? (F)"=TRUE, "error in (no error)"=w1187, "Message"="Write bit pattern to FVIR and LDO", "Message Queue"=w1185) -> ("error out"=w1186:errorcluster)  [unwired: 6 in, 1 out]
      }
      frame "Output_Flow_Target_FVIR" {
        n185 = Variant To Data(error in=w1213, type=0.0 ("Numeric"), Variant=w1212) -> (data=w1216:dbl, error out=w1217:errorcluster)
        n186 = call "UTILITY Modbus 32bit Number to 16bit Array.vi"("error in"=w1217, "32-bit IEEE 754"=w1216) -> ("error out"=w1219:errorcluster, "U16 Array Representation"=w1218:u16[])  [unwired: 8 in]
        n187 = call-dynamic "Write Multiple Holding Registers.vi"("error in"=w1219, "registers to write"=w1218, "starting address"=u16 55 ("address"), "Modbus master in"=w1211) -> ("error out"=w1208:errorcluster, "Modbus master out"=w1210:refnum<class "Modbus Master.lvclass">)  [unwired: 6 in]
        n188 = call-poly "Enqueue Message.vi"("Priority Message? (F)"=TRUE, "error in (no error)"=w1208, "Message"="Write bit pattern to FVIR and LDO", "Message Queue"=w1206) -> ("error out"=w1207:errorcluster)  [unwired: 6 in, 1 out]
      }
      frame "MannequinGoToHomePos" {
        n189 = Replace Array Subset(array=w1234, new element=TRUE ("new element/subarray"), index=10) -> (w1233:bool[])
        n190 = call-poly "Enqueue Message.vi"("Priority Message? (F)"=TRUE, "error in (no error)"=w1236, "Message"="Write bit pattern to FVIR and LDO", "Message Queue"=w1231) -> ("error out"=w1224:errorcluster)  [unwired: 6 in, 1 out]
      }
      frame "MannequinGoToHomePosClear" {
        n191 = Replace Array Subset(array=w1247, new element=FALSE ("new element/subarray"), index=10) -> (w1246:bool[])
        n192 = call-poly "Enqueue Message.vi"("Priority Message? (F)"=TRUE, "error in (no error)"=w1249, "Message"="Write bit pattern to FVIR and LDO", "Message Queue"=w1253) -> ("error out"=w1252:errorcluster)  [unwired: 6 in, 1 out]
      }
      frame "MannequinGoToWorkPos" {
        n193 = Replace Array Subset(array=w1264, new element=TRUE ("new element/subarray"), index=9) -> (w1263:bool[])
        n194 = call-poly "Enqueue Message.vi"("Priority Message? (F)"=TRUE, "error in (no error)"=w1266, "Message"="Write bit pattern to FVIR and LDO", "Message Queue"=w1261) -> ("error out"=w1254:errorcluster)  [unwired: 6 in, 1 out]
      }
      frame "MannequinGoToWorkPosClear" {
        n195 = Replace Array Subset(array=w1277, new element=FALSE ("new element/subarray"), index=9) -> (w1276:bool[])
        n196 = call-poly "Enqueue Message.vi"("Priority Message? (F)"=TRUE, "error in (no error)"=w1279, "Message"="Write bit pattern to FVIR and LDO", "Message Queue"=w1283) -> ("error out"=w1282:errorcluster)  [unwired: 6 in, 1 out]
      }
      frame "SpillCanGoToHomePos" {
        n197 = Replace Array Subset(array=w1294, new element=TRUE ("new element/subarray"), index=11) -> (w1293:bool[])
        n198 = call-poly "Enqueue Message.vi"("Priority Message? (F)"=TRUE, "error in (no error)"=w1296, "Message"="Write bit pattern to FVIR and LDO", "Message Queue"=w1291) -> ("error out"=w1284:errorcluster)  [unwired: 6 in, 1 out]
      }
      frame "SpillCanGoToHomePosClear" {
        n199 = Replace Array Subset(array=w1307, new element=FALSE ("new element/subarray"), index=11) -> (w1306:bool[])
        n200 = call-poly "Enqueue Message.vi"("Priority Message? (F)"=TRUE, "error in (no error)"=w1309, "Message"="Write bit pattern to FVIR and LDO", "Message Queue"=w1313) -> ("error out"=w1312:errorcluster)  [unwired: 6 in, 1 out]
      }
      frame "SpillCanGoToWorkPos" {
        n201 = Replace Array Subset(array=w1324, new element=TRUE ("new element/subarray"), index=12) -> (w1323:bool[])
        n202 = call-poly "Enqueue Message.vi"("Priority Message? (F)"=TRUE, "error in (no error)"=w1326, "Message"="Write bit pattern to FVIR and LDO", "Message Queue"=w1321) -> ("error out"=w1314:errorcluster)  [unwired: 6 in, 1 out]
      }
      frame "SpillCanGoToWorkPosClear" {
        n203 = Replace Array Subset(array=w1337, new element=FALSE ("new element/subarray"), index=12) -> (w1336:bool[])
        n204 = call-poly "Enqueue Message.vi"("Priority Message? (F)"=TRUE, "error in (no error)"=w1339, "Message"="Write bit pattern to FVIR and LDO", "Message Queue"=w1343) -> ("error out"=w1342:errorcluster)  [unwired: 6 in, 1 out]
      }
      frame "ResetFlowMeter_ON_FVIR" {
        n205 = call-poly "Enqueue Message.vi"("Priority Message? (F)"=TRUE, "error in (no error)"=w1355, "Message"="Write bit pattern to FVIR and LDO", "Message Queue"=w1356) -> ("error out"=w1354:errorcluster)  [unwired: 6 in, 1 out]
        n206 = Replace Array Subset(array=w1347, new element=TRUE ("new element/subarray"), index=13) -> (w1346:bool[])
      }
      frame "ResetFlowMeter_OFF_FVIR" {
        n207 = call-poly "Enqueue Message.vi"("Priority Message? (F)"=TRUE, "error in (no error)"=w1369, "Message"="Write bit pattern to FVIR and LDO", "Message Queue"=w1368) -> ("error out"=w1367:errorcluster)  [unwired: 6 in, 1 out]
        n208 = Replace Array Subset(array=w1362, new element=FALSE ("new element/subarray"), index=13) -> (w1361:bool[])
      }
      frame "Water_Heater_Status_ON_FVIR" {
        n209 = Replace Array Subset(array=w1382, new element=TRUE ("new element/subarray"), index=14) -> (w1381:bool[])
        n210 = call-poly "Enqueue Message.vi"("Priority Message? (F)"=TRUE, "error in (no error)"=w1384, "Message"="Write bit pattern to FVIR and LDO", "Message Queue"=w1388) -> ("error out"=w1387:errorcluster)  [unwired: 6 in, 1 out]
      }
      frame "Water_Heater_Status_OFF_FVIR" {
        n211 = Replace Array Subset(array=w1397, new element=FALSE ("new element/subarray"), index=14) -> (w1396:bool[])
        n212 = call-poly "Enqueue Message.vi"("Priority Message? (F)"=TRUE, "error in (no error)"=w1399, "Message"="Write bit pattern to FVIR and LDO", "Message Queue"=w1403) -> ("error out"=w1402:errorcluster)  [unwired: 6 in, 1 out]
      }
      frame "PID_Selector_OFF_FVIR" {
        n213 = Replace Array Subset(array=w1408, new element=FALSE ("new element/subarray"), index=15) -> (w1407:bool[])
        n214 = call-poly "Enqueue Message.vi"("Priority Message? (F)"=TRUE, "error in (no error)"=w1412, "Message"="Write bit pattern to FVIR and LDO", "Message Queue"=w1413) -> ("error out"=w1411:errorcluster)  [unwired: 6 in, 1 out]
      }
      frame "TestCase1Winter" {
        # "Writing to PLC with value 1 at address 7"
        n215 = call-dynamic "Write Single Holding Register.vi"("error in"=w1434, "register to write"=u16 1, "address"=u16 7 ("starting address"), "Modbus master in"=w1432) -> ("error out"=w1428:errorcluster, "Modbus master out"=w1433:refnum<class "Modbus Master.lvclass">)  [unwired: 6 in]
        n216 = call-poly "Enqueue Message.vi"("Priority Message? (F)"=TRUE, "error in (no error)"=w1428, "Message"="Write bit pattern to FVIR and LDO", "Message Queue"=w1429) -> ("error out"=w1426:errorcluster)  [unwired: 6 in, 1 out]
      }
      frame "TestCase1Summer" {
        # "Writing to PLC with value 2 at address 7"
        n217 = call-dynamic "Write Single Holding Register.vi"("error in"=w1450, "register to write"=u16 2, "address"=u16 7 ("starting address"), "Modbus master in"=w1448) -> ("error out"=w1444:errorcluster, "Modbus master out"=w1449:refnum<class "Modbus Master.lvclass">)  [unwired: 6 in]
        n218 = call-poly "Enqueue Message.vi"("Priority Message? (F)"=TRUE, "error in (no error)"=w1444, "Message"="Write bit pattern to FVIR and LDO", "Message Queue"=w1445) -> ("error out"=w1442:errorcluster)  [unwired: 6 in, 1 out]
      }
      frame "TestCase2Winter" {
        # "Writing to PLC with value 3 at address 7"
        n219 = call-dynamic "Write Single Holding Register.vi"("error in"=w1466, "register to write"=u16 3, "address"=u16 7 ("starting address"), "Modbus master in"=w1464) -> ("error out"=w1460:errorcluster, "Modbus master out"=w1465:refnum<class "Modbus Master.lvclass">)  [unwired: 6 in]
        n220 = call-poly "Enqueue Message.vi"("Priority Message? (F)"=TRUE, "error in (no error)"=w1460, "Message"="Write bit pattern to FVIR and LDO", "Message Queue"=w1461) -> ("error out"=w1458:errorcluster)  [unwired: 6 in, 1 out]
      }
      frame "TestCase2Summer" {
        # "Writing to PLC with value 4 at address 7"
        n221 = call-dynamic "Write Single Holding Register.vi"("error in"=w1482, "register to write"=u16 4, "address"=u16 7 ("starting address"), "Modbus master in"=w1480) -> ("error out"=w1476:errorcluster, "Modbus master out"=w1481:refnum<class "Modbus Master.lvclass">)  [unwired: 6 in]
        n222 = call-poly "Enqueue Message.vi"("Priority Message? (F)"=TRUE, "error in (no error)"=w1476, "Message"="Write bit pattern to FVIR and LDO", "Message Queue"=w1477) -> ("error out"=w1474:errorcluster)  [unwired: 6 in, 1 out]
      }
      frame "TestCase3Winter" {
        # "Writing to PLC with value 5 at address 7"
        n223 = call-dynamic "Write Single Holding Register.vi"("error in"=w1498, "register to write"=u16 5, "address"=u16 7 ("starting address"), "Modbus master in"=w1496) -> ("error out"=w1492:errorcluster, "Modbus master out"=w1497:refnum<class "Modbus Master.lvclass">)  [unwired: 6 in]
        n224 = call-poly "Enqueue Message.vi"("Priority Message? (F)"=TRUE, "error in (no error)"=w1492, "Message"="Write bit pattern to FVIR and LDO", "Message Queue"=w1493) -> ("error out"=w1490:errorcluster)  [unwired: 6 in, 1 out]
      }
      frame "TestCase3Summer" {
        # "Writing to PLC with value 6 at address 7"
        n225 = call-dynamic "Write Single Holding Register.vi"("error in"=w1514, "register to write"=u16 6, "address"=u16 7 ("starting address"), "Modbus master in"=w1512) -> ("error out"=w1508:errorcluster, "Modbus master out"=w1513:refnum<class "Modbus Master.lvclass">)  [unwired: 6 in]
        n226 = call-poly "Enqueue Message.vi"("Priority Message? (F)"=TRUE, "error in (no error)"=w1508, "Message"="Write bit pattern to FVIR and LDO", "Message Queue"=w1509) -> ("error out"=w1506:errorcluster)  [unwired: 6 in, 1 out]
      }
      frame "TestCase4Winter" {
        # "Writing to PLC with value 7 at address 7"
        n227 = call-dynamic "Write Single Holding Register.vi"("error in"=w1522, "register to write"=u16 7, "address"=u16 7 ("starting address"), "Modbus master in"=w1529) -> ("error out"=w1525:errorcluster, "Modbus master out"=w1530:refnum<class "Modbus Master.lvclass">)  [unwired: 6 in]
        n228 = call-poly "Enqueue Message.vi"("Priority Message? (F)"=TRUE, "error in (no error)"=w1525, "Message"="Write bit pattern to FVIR and LDO", "Message Queue"=w1526) -> ("error out"=w1523:errorcluster)  [unwired: 6 in, 1 out]
      }
      frame "TestCase4Summer" {
        # "Writing to PLC with value 8 at address 7"
        n229 = call-dynamic "Write Single Holding Register.vi"("error in"=w1546, "register to write"=u16 8, "address"=u16 7 ("starting address"), "Modbus master in"=w1544) -> ("error out"=w1540:errorcluster, "Modbus master out"=w1545:refnum<class "Modbus Master.lvclass">)  [unwired: 6 in]
        n230 = call-poly "Enqueue Message.vi"("Priority Message? (F)"=TRUE, "error in (no error)"=w1540, "Message"="Write bit pattern to FVIR and LDO", "Message Queue"=w1541) -> ("error out"=w1538:errorcluster)  [unwired: 6 in, 1 out]
      }
    }
    n231 = case shown="True" "Read States" {
      tunnel: w21 -> [w39 w48]
      tunnel: [w39 w41] -> w20
      tunnel: w12 -> [_ w44]
      frame False {
      }
      frame True {
        n232 = Get Queue Status(queue=w44, return elements? (F)=TRUE) -> (elements=w46:T1[])  [unwired: 1 in, 7 out]
        "elements" <- w46
        n233 = Array Size(array=w46) -> (size(s)=→"size(s)":i32)
        n234 = Index Array(array=w46) -> (element=w47:T1)  [unwired: 1 in]
        n235 = Unbundle By Name(w47) -> ("Message"=w42:string)
        "Current State" <- w42
        n236 = Build Array (concatenate)(w48, w42) -> (w41:string[])
        n237 = Reverse 1D Array(array=w41) -> (reversed array=→"States":string[])
      }
    }
    n238 = Wait Until Next ms Multiple(millisecond multiple=w16) -> ()  [unwired: 1 out]
    n239 = call "Error Handler - Message Handling Loop.vi"("error in (no error)"=w15, "Message Queue"=w11) -> ("dup error in"=w36:errorcluster)  [unwired: 8 in, 1 out]
    "Loop Count" <- w22
  }
  "error out" <- w1
